vi "Motors Bk.vi"(2 "Motors Visa Ref":refnum<visa-resource-name>="COM7") -> ()   [LabVIEW 2010]
panel:
  in  "Cluster":T1
  in  "Y Speed (mm/s)":dbl=1.0 min=0.0
  in  "Delta Y (mm)":dbl=1.0
  in  "Theta Speed (deg/s)":dbl=1.0 min=0.0
  in  "Delta Theta (deg)":dbl=1.0
  in  "(mm/s)":dbl min=0.4
  in  "(mm/s) 3":dbl min=0.4
  in  "(mm/s) 2":dbl min=4.0
  in  "(degrees/s)":dbl min=8.0
  in  "X Set Slew Speed":bool
  in  "Y Set Slew Speed":bool
  in  "Z Set Slew Speed":bool
  in  "Theta Set Slew Speed":bool
  in  "Go To Saved Position":bool
  in  "Defined Positions":i32(listbox)
  in  "Steps to deactivate hard limit after finding datums":dbl=500.0
  out "Loop i":i32
types:
  T1 = cluster{"Stop X?":refnum<vi>, "Stop Y?":refnum<vi>, "Stop Z?":refnum<vi>, "Stop Theta?":refnum<vi>, "Backlash?":refnum<vi>, "Backlash X":refnum<vi>, "Backlash Y":refnum<vi>, "Backlash Z":refnum<vi>, "Backlash Theta":refnum<vi>, "Manual IO?":refnum<vi>, "Manual Communication is Active\n(Close Before Ending Program)":refnum<vi>, "Reset Motors?":refnum<vi>, "Set Jogger?":refnum<vi>, "Normal":refnum<vi>, "Fast":refnum<vi>, "Jogger Axis":refnum<vi>, "Redefine Origin as Current Location?":refnum<vi>, "Save Current Motor Parameters?":refnum<vi>, "Find Datums Nearest Hard Limits?":refnum<vi>, "Saved Limits":refnum<vi>, "Use Datums Nearest Hard Limits to Reset Origin?":refnum<vi>, "X Go?":refnum<vi>, "Y Go?":refnum<vi>, "Z Go?":refnum<vi>, "Theta Go?":refnum<vi>, "Jog-Mode":refnum<vi>, "x+?":refnum<vi>, "x-?":refnum<vi>, "y+?":refnum<vi>, "y-?":refnum<vi>, "z+?":refnum<vi>, "z-?":refnum<vi>, "theta+?":refnum<vi>, "theta-?":refnum<vi>, "X Set Slew Speed?":refnum<vi>, "(mm/s)":refnum<vi>, "Y Set Slew Speed?":refnum<vi>, "(mm/s)":refnum<vi>, "Z Set Slew Speed?":refnum<vi>, "(mm/s)":refnum<vi>, "Theta Set Slew Speed?":refnum<vi>, "(degrees/s)":refnum<vi>, "Go To Saved Position?":refnum<vi>, "Defined Positions":refnum<vi>, "Need to Update Motor Parameters":refnum<vi>, "X Jogger Normal Speed":refnum<vi>, "X Jogger Fast Speed":refnum<vi>, "Y Jogger Normal Speed":refnum<vi>, "Y Jogger Fast Speed":refnum<vi>, "Z Jogger Normal Speed":refnum<vi>, "Z Jogger Fast Speed":refnum<vi>, "Theta Jogger Normal Speed":refnum<vi>, "Theta Jogger Fast Speed":refnum<vi>, "X Moving":refnum<vi>, "Y Moving":refnum<vi>, "Z Moving":refnum<vi>, "Theta Moving":refnum<vi>, "X Slew Speed (mm or degree/s)":refnum<vi>, "Y Slew Speed (mm or degree/s)":refnum<vi>, "Z Slew Speed (mm or degree/s)":refnum<vi>, "Theta Slew Speed (mm or degree/s)":refnum<vi>, "X-Axis (mm)":refnum<vi>, "Y-Axis (mm)":refnum<vi>, "Z-Axis (mm)":refnum<vi>, "Theta (deg)":refnum<vi>, "X Multiplier":refnum<vi>, "Y Multiplier":refnum<vi>, "Z Multiplier":refnum<vi>, "Theta Multiplier":refnum<vi>, "Motors Online":refnum<vi>, "Motors Status":refnum<vi>, "Status X":refnum<vi>, "Status Y":refnum<vi>, "Status Z":refnum<vi>, "Status Theta":refnum<vi>, "Motors error":refnum<vi>, "QUIT":refnum<vi>, "EMERGENCY":refnum<vi>, "X Go To":refnum<vi>, "Y Go To":refnum<vi>, "Z Go To":refnum<vi>, "Theta Go To":refnum<vi>, "Delta X (mm)":refnum<vi>, "Delta Y (mm)":refnum<vi>, "Delta Z (mm)":refnum<vi>, "Delta Theta (deg)":refnum<vi>, "X Speed (mm/s)":refnum<vi>, "Y Speed (mm/s)":refnum<vi>, "Z Speed (mm/s)":refnum<vi>, "Theta Speed (deg/s)":refnum<vi>, "x+":refnum<vi>, "x-":refnum<vi>, "y+":refnum<vi>, "y-":refnum<vi>, "z+":refnum<vi>, "z-":refnum<vi>, "theta+":refnum<vi>, "theta-":refnum<vi>}
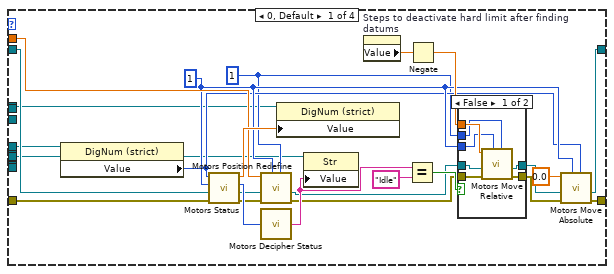
[diagram p4: hidden frame]
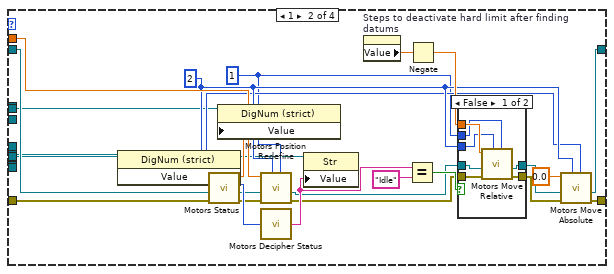
[diagram p6: hidden frame]
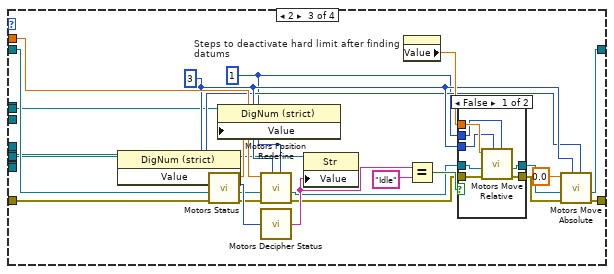
[diagram p8: hidden frame]
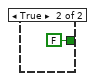
[diagram p12: hidden frame]
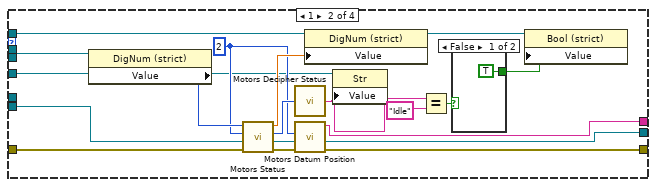
[diagram p13: hidden frame]
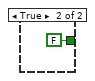
[diagram p14: hidden frame]
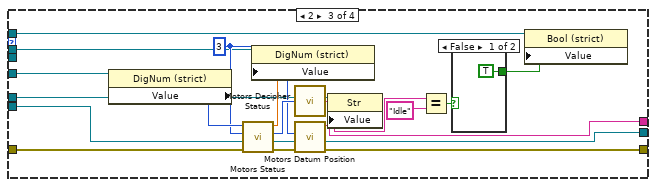
[diagram p15: hidden frame]
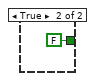
[diagram p16: hidden frame]
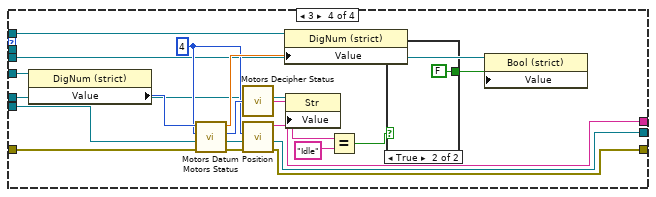
[diagram p17: hidden frame]
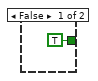
[diagram p18: hidden frame]
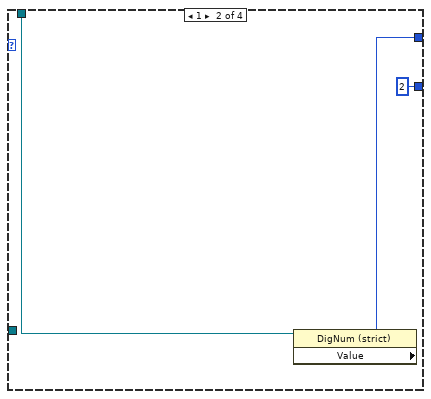
[diagram p19: hidden frame]
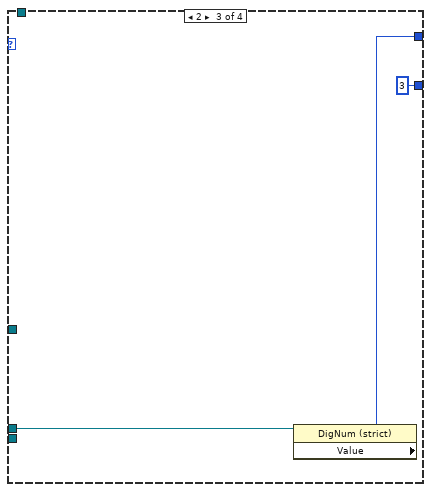
[diagram p20: hidden frame]
diagram:
  n1 = Unbundle("Cluster") -> ("Stop X?"=w69:refnum<vi>, "Stop Y?"=w68:refnum<vi>, "Stop Z?"=w67:refnum<vi>, "Stop Theta?"=w66:refnum<vi>, "Backlash?"=w65:refnum<vi>, "Backlash X"=w64:refnum<vi>, "Backlash Y"=w63:refnum<vi>, "Backlash Z"=w62:refnum<vi>, "Backlash Theta"=w61:refnum<vi>, "Manual IO?"=w60:refnum<vi>, "Manual Communication is Active\n(Close Before Ending Program)"=w53:refnum<vi>, "Reset Motors?"=w51:refnum<vi>, "Set Jogger?"=w50:refnum<vi>, "Normal"=w48:refnum<vi>, "Fast"=w47:refnum<vi>, "Jogger Axis"=w49:refnum<vi>, "Redefine Origin as Current Location?"=w46:refnum<vi>, "Save Current Motor Parameters?"=w45:refnum<vi>, "Find Datums Nearest Hard Limits?"=w44:refnum<vi>, "Saved Limits"=w43:refnum<vi>, "Use Datums Nearest Hard Limits to Reset Origin?"=w42:refnum<vi>, "X Go?"=w32:refnum<vi>, "Y Go?"=w29:refnum<vi>, "Z Go?"=w28:refnum<vi>, "Theta Go?"=w25:refnum<vi>, "Jog-Mode"=w22:refnum<vi>, "x+?"=w14:refnum<vi>, "x-?"=w15:refnum<vi>, "y+?"=w13:refnum<vi>, "y-?"=w12:refnum<vi>, "Need to Update Motor Parameters"=w34:refnum<vi>, "X Moving"=w21:refnum<vi>, "Y Moving"=w3:refnum<vi>, "Z Moving"=w41:refnum<vi>, "Theta Moving"=w40:refnum<vi>, "X-Axis (mm)"=w17:refnum<vi>, "Y-Axis (mm)"=w10:refnum<vi>, "Z-Axis (mm)"=w39:refnum<vi>, "Theta (deg)"=w37:refnum<vi>, "X Multiplier"=w19:refnum<vi>, "Y Multiplier"=w1:refnum<vi>, "Z Multiplier"=w27:refnum<vi>, "Theta Multiplier"=w24:refnum<vi>, "Motors Online"=w54:refnum<vi>, "Motors Status"=w56:refnum<vi>, "Status X"=w16:refnum<vi>, "Status Y"=w4:refnum<vi>, "Status Z"=w38:refnum<vi>, "Status Theta"=w36:refnum<vi>, "Motors error"=w59:refnum<vi>, "QUIT"=w58:refnum<vi>, "EMERGENCY"=w52:refnum<vi>, "X Go To"=w31:refnum<vi>, "Y Go To"=w30:refnum<vi>, "Z Go To"=w26:refnum<vi>, "Theta Go To"=w23:refnum<vi>, "Delta X (mm)"=w20:refnum<vi>, "Delta Y (mm)"=w2:refnum<vi>, "X Speed (mm/s)"=w18:refnum<vi>, "Y Speed (mm/s)"=w11:refnum<vi>, "x+"=w8:refnum<vi>, "x-"=w7:refnum<vi>, "y+"=w6:refnum<vi>, "y-"=w5:refnum<vi>)  [unwired: 34 out]
  n2 = property on="Property Node" class="Bool (strict)"(reference=w34, "Value"=TRUE) -> (reference out=w35:refnum<vi>)  [unwired: 1 in, 1 out]
  n3 = call "Motors Open.vi"("VISA in"="Motors Visa Ref") -> ("error out"=w73:errorcluster, "VISA out"=w70:refnum<visa-resource-name>)  [unwired: 1 in]
  n4 = call <vilib>:"Simple Error Handler.vi"("error in (no error)"=w73) -> ("error?"=w72:bool, "error out"=w74:errorcluster)  [unwired: 4 in, 3 out]
  n5 = property on="Property Node" class="Str"(reference=w56, "Value"="Opening Communications") -> (reference out=w57:refnum<vi>)  [unwired: 1 in, 1 out]
  n6 = property on="Property Node" class="Clust (strict)"(reference=w59, "Value"=w74) -> ()  [unwired: 1 in, 2 out]
  n7 = Not(x=w72) -> (.not. x?=w71:bool)
  n8 = case shown="True" w71 {
    tunnel: w57 -> [_ w164]
    tunnel: w70 -> [_ w163]
    tunnel: w59 -> [_ w162]
    tunnel: w58 -> [_ w161]
    tunnel: w69 -> [_ w160]
    tunnel: w68 -> [_ w159]
    tunnel: w67 -> [_ w158]
    tunnel: w66 -> [_ w157]
    tunnel: w65 -> [_ w156]
    tunnel: w64 -> [_ w155]
    tunnel: w63 -> [_ w154]
    tunnel: w62 -> [_ w153]
    tunnel: w61 -> [_ w152]
    tunnel: w60 -> [_ w151]
    tunnel: w53 -> [_ w150]
    tunnel: w52 -> [_ w149]
    tunnel: w51 -> [_ w148]
    tunnel: w50 -> [_ w147]
    tunnel: w49 -> [_ w146]
    tunnel: w19 -> [_ w145]
    tunnel: w1 -> [_ w144]
    tunnel: w27 -> [_ w143]
    tunnel: w24 -> [_ w142]
    tunnel: w35 -> [_ w141]
    tunnel: w48 -> [_ w140]
    tunnel: w47 -> [_ w139]
    tunnel: w46 -> [_ w138]
    tunnel: w45 -> [_ w137]
    tunnel: w44 -> [_ w136]
    tunnel: w19 -> [_ w134]
    tunnel: w17 -> [_ w133]
    tunnel: w16 -> [_ w132]
    tunnel: w21 -> [_ w131]
    tunnel: w43 -> [_ w130]
    tunnel: w42 -> [_ w129]
    tunnel: w3 -> [_ w128]
    tunnel: w41 -> [_ w127]
    tunnel: w40 -> [_ w126]
    tunnel: w19 -> [_ w125]
    tunnel: w1 -> [_ w124]
    tunnel: w27 -> [_ w123]
    tunnel: w24 -> [_ w122]
    tunnel: w17 -> [_ w121]
    tunnel: w10 -> [_ w120]
    tunnel: w39 -> [_ w119]
    tunnel: w16 -> [_ w118]
    tunnel: w4 -> [_ w117]
    tunnel: w38 -> [_ w116]
    tunnel: w37 -> [_ w115]
    tunnel: w36 -> [_ w114]
    tunnel: w32 -> [_ w113]
    tunnel: w19 -> [_ w112]
    tunnel: w31 -> [_ w111]
    tunnel: w1 -> [_ w110]
    tunnel: w30 -> [_ w109]
    tunnel: w29 -> [_ w108]
    tunnel: w28 -> [_ w107]
    tunnel: w27 -> [_ w106]
    tunnel: w26 -> [_ w105]
    tunnel: w25 -> [_ w104]
    tunnel: w24 -> [_ w103]
    tunnel: w23 -> [_ w102]
    tunnel: w15 -> [_ w101]
    tunnel: w22 -> [_ w100]
    tunnel: w21 -> [_ w99]
    tunnel: w20 -> [_ w98]
    tunnel: w19 -> [_ w97]
    tunnel: w18 -> [_ w96]
    tunnel: w17 -> [_ w95]
    tunnel: w14 -> [_ w94]
    tunnel: w15 -> [_ w93]
    tunnel: w16 -> [_ w92]
    tunnel: w15 -> [_ w91]
    tunnel: w14 -> [_ w90]
    tunnel: w14 -> [_ w89]
    tunnel: w13 -> [_ w88]
    tunnel: w12 -> [_ w87]
    tunnel: w1 -> [_ w86]
    tunnel: w11 -> [_ w85]
    tunnel: w10 -> [_ w84]
    tunnel: w8 -> [_ w83]
    tunnel: w7 -> [_ w82]
    tunnel: w6 -> [_ w81]
    tunnel: w5 -> [_ w80]
    tunnel: w4 -> [_ w79]
    tunnel: w3 -> [_ w78]
    tunnel: w2 -> [_ w77]
    tunnel: w1 -> [_ w76]
    frame False {
    }
    frame True {
      n9 = property on="Property Node" class="Str"(reference=w164, "Value"="Running") -> (reference out=w135:refnum<vi>)  [unwired: 1 in, 1 out]
      n10 = while {
        shift-right: _ -> [_]
        shift-left: w163 -> [w368]
        tunnel: w162 -> [w370]
        tunnel: w161 -> [w292]
        tunnel: w160 -> [w291]
        tunnel: w159 -> [w289]
        tunnel: w158 -> [w287]
        tunnel: w157 -> [w285]
        tunnel: w156 -> [w283]
        tunnel: w155 -> [w281]
        tunnel: w154 -> [w280]
        tunnel: w153 -> [w279]
        tunnel: w152 -> [w278]
        tunnel: w151 -> [w277]
        tunnel: w150 -> [w275]
        tunnel: w149 -> [w274]
        tunnel: w148 -> [w273]
        tunnel: w147 -> [w271]
        tunnel: w146 -> [w268]
        tunnel: w145 -> [w267]
        tunnel: w144 -> [w266]
        tunnel: w143 -> [w265]
        tunnel: w142 -> [w264]
        tunnel: w141 -> [w263]
        tunnel: w140 -> [w262]
        tunnel: w139 -> [w261]
        tunnel: w138 -> [w259]
        tunnel: w137 -> [w258]
        tunnel: w136 -> [w256]
        tunnel: w135 -> [w255]
        tunnel: w134 -> [w254]
        tunnel: w133 -> [w253]
        tunnel: w132 -> [w252]
        tunnel: w131 -> [w251]
        tunnel: w130 -> [w250]
        tunnel: w129 -> [w229]
        tunnel: w128 -> [w248]
        tunnel: w127 -> [w247]
        tunnel: w126 -> [w246]
        tunnel: w125 -> [w243]
        tunnel: w124 -> [w242]
        tunnel: w123 -> [w241]
        tunnel: w122 -> [w240]
        tunnel: w121 -> [w239]
        tunnel: w120 -> [w238]
        tunnel: w119 -> [w237]
        tunnel: w118 -> [w236]
        tunnel: w117 -> [w235]
        tunnel: w116 -> [w234]
        tunnel: w115 -> [w233]
        tunnel: w114 -> [w232]
        tunnel: w113 -> [w230]
        tunnel: w112 -> [w214]
        tunnel: w111 -> [w213]
        tunnel: w110 -> [w212]
        tunnel: w109 -> [w211]
        tunnel: w108 -> [w209]
        tunnel: w107 -> [w206]
        tunnel: w106 -> [w204]
        tunnel: w105 -> [w203]
        tunnel: w104 -> [w201]
        tunnel: w103 -> [w197]
        tunnel: w102 -> [w199]
        tunnel: w101 -> [w198]
        tunnel: w100 -> [w195]
        tunnel: w99 -> [w194]
        tunnel: w98 -> [w193]
        tunnel: w97 -> [w192]
        tunnel: w96 -> [w191]
        tunnel: w95 -> [w190]
        tunnel: w94 -> [w189]
        tunnel: w93 -> [w188]
        tunnel: w92 -> [w187]
        tunnel: w91 -> [w186]
        tunnel: w90 -> [w185]
        tunnel: w89 -> [w184]
        tunnel: w88 -> [w183]
        tunnel: w87 -> [w182]
        tunnel: w86 -> [w181]
        tunnel: w85 -> [w180]
        tunnel: w84 -> [w179]
        tunnel: w83 -> [w175]
        tunnel: w82 -> [w174]
        tunnel: w81 -> [w173]
        tunnel: w80 -> [w172]
        tunnel: w79 -> [w171]
        tunnel: w78 -> [w168]
        tunnel: w77 -> [w167]
        tunnel: w76 -> [w166]
        i -> [w293]
        stop <- w371 stop-if-true
        # "This loop contains all of the code that has to communicate directly with the manipulator motor controllers.  They are arranged linearly to ensure multiple serial I/O's are never attempted simultaneously.  Note that this loop executes very slowly (each serial I/O takes about 1/20 sec)."
        n11 = property on="Property Node" class="Bool (strict)"(reference=w183) -> (reference out=w169:refnum<vi>, "Value"=w307:bool)  [unwired: 1 in, 1 out]
        n12 = property on="Property Node" class="Bool (strict)"(reference=w182) -> (reference out=w170:refnum<vi>, "Value"=w308:bool)  [unwired: 1 in, 1 out]
        n13 = Or(x=w307, y=w308) -> (x .or. y?=w338:bool)
        n14 = property on="Property Node" class="Bool (strict)"(reference=w198) -> (reference out=w177:refnum<vi>, "Value"=w311:bool)  [unwired: 1 in, 1 out]
        n15 = property on="Property Node" class="Bool (strict)"(reference=w185) -> (reference out=w176:refnum<vi>, "Value"=w312:bool)  [unwired: 1 in, 1 out]
        n16 = property on="Property Node" class="Bool (strict)"(reference=w195) -> ("Value"=w196:bool)  [unwired: 1 in, 2 out]
        n17 = property on="Property Node" class="Bool (strict)"(reference=w230) -> (reference out=w178:refnum<vi>, "Value"=w231:bool)  [unwired: 1 in, 1 out]
        n18 = property on="Property Node" class="Bool (strict)"(reference=w292) -> ("Value"=w371:bool)  [unwired: 1 in, 2 out]
        n19 = Or(x=w312, y=w311) -> (x .or. y?=w344:bool)
        n20 = property on="Property Node" class="Bool (strict)"(reference=w291) -> (reference out=w215:refnum<vi>, "Value"=w290:bool)  [unwired: 1 in, 1 out]
        n21 = property on="Property Node" class="DigNum (strict)" props=["Value"]() -> ()  [unwired: 2 in, 3 out]
        n22 = property on="Property Node" class="Bool (strict)"(reference=w289) -> (reference out=w216:refnum<vi>, "Value"=w288:bool)  [unwired: 1 in, 1 out]
        n23 = property on="Property Node" class="Clust (strict)"(reference=w370) -> ("Value"=w369:errorcluster)  [unwired: 1 in, 2 out]
        n24 = property on="Property Node" class="Bool (strict)"(reference=w287) -> (reference out=w217:refnum<vi>, "Value"=w286:bool)  [unwired: 1 in, 1 out]
        n25 = property on="Property Node" class="Bool (strict)"(reference=w209) -> (reference out=w208:refnum<vi>, "Value"=w210:bool)  [unwired: 1 in, 1 out]
        n26 = case shown="True" w290 {
          tunnel: w369 -> [w1519 w1527]
          tunnel: w368 -> [w1520 w1526]
          tunnel: [w1520 w1524] -> w362
          tunnel: [w1519 w1523] -> w363
          tunnel: w215 -> [_ w1521]
          frame False {
          }
          frame True {
            n27 = call "Motors Stop.vi"("error in"=w1527, "Axis"=1, "VISA in"=w1526) -> ("error out"=w1523:errorcluster, "VISA out"=w1524:refnum<visa-resource-name>)
            n28 = property on="Property Node" class="Bool (strict)"(reference=w1521, "Value"=FALSE) -> ()  [unwired: 1 in, 2 out]
          }
        }
        n29 = property on="Property Node" class="Bool (strict)"(reference=w206) -> (reference out=w205:refnum<vi>, "Value"=w207:bool)  [unwired: 1 in, 1 out]
        n30 = case shown="True" w288 {
          tunnel: w363 -> [w1510 w1518]
          tunnel: w362 -> [w1511 w1517]
          tunnel: [w1511 w1515] -> w364
          tunnel: [w1510 w1514] -> w365
          tunnel: w216 -> [_ w1512]
          frame False {
          }
          frame True {
            n31 = call "Motors Stop.vi"("error in"=w1518, "Axis"=2, "VISA in"=w1517) -> ("error out"=w1514:errorcluster, "VISA out"=w1515:refnum<visa-resource-name>)
            n32 = property on="Property Node" class="Bool (strict)"(reference=w1512, "Value"=FALSE) -> ()  [unwired: 1 in, 2 out]
          }
        }
        n33 = property on="Property Node" class="Bool (strict)"(reference=w285) -> (reference out=w218:refnum<vi>, "Value"=w284:bool)  [unwired: 1 in, 1 out]
        n34 = case shown="True" w286 {
          tunnel: w365 -> [w1501 w1509]
          tunnel: w364 -> [w1502 w1508]
          tunnel: [w1502 w1506] -> w366
          tunnel: [w1501 w1505] -> w367
          tunnel: w217 -> [_ w1503]
          frame False {
          }
          frame True {
            n35 = call "Motors Stop.vi"("error in"=w1509, "Axis"=3, "VISA in"=w1508) -> ("error out"=w1505:errorcluster, "VISA out"=w1506:refnum<visa-resource-name>)
            n36 = property on="Property Node" class="Bool (strict)"(reference=w1503, "Value"=FALSE) -> ()  [unwired: 1 in, 2 out]
          }
        }
        n37 = property on="Property Node" class="Bool (strict)"(reference=w283) -> (reference out=w219:refnum<vi>, "Value"=w282:bool)  [unwired: 1 in, 1 out]
        n38 = property on="Property Node" class="Bool (strict)"(reference=w201) -> (reference out=w200:refnum<vi>, "Value"=w202:bool)  [unwired: 1 in, 1 out]
        n39 = case shown="True" w284 {
          tunnel: w367 -> [w1492 w1500]
          tunnel: w366 -> [w1493 w1499]
          tunnel: [w1493 w1497] -> w360
          tunnel: [w1492 w1496] -> w361
          tunnel: w218 -> [_ w1494]
          frame False {
          }
          frame True {
            n40 = property on="Property Node" class="Bool (strict)"(reference=w1494, "Value"=FALSE) -> ()  [unwired: 1 in, 2 out]
            n41 = call "Motors Stop.vi"("error in"=w1500, "Axis"=4, "VISA in"=w1499) -> ("error out"=w1496:errorcluster, "VISA out"=w1497:refnum<visa-resource-name>)
          }
        }
        n42 = case shown="True" w282 {
          tunnel: w360 -> [w1477 w1491]
          tunnel: [w1477 w1490] -> w359
          tunnel: [w1476 w1489] -> w358
          tunnel: w361 -> [w1476 w1488]
          tunnel: w281 -> [_ w1487]
          tunnel: w280 -> [_ w1485]
          tunnel: w279 -> [_ w1483]
          tunnel: w278 -> [_ w1481]
          tunnel: w219 -> [_ w1478]
          frame False {
          }
          frame True {
            n43 = property on="Property Node" class="DigNum (strict)"(reference=w1483) -> ("Value"=w1482:u32)  [unwired: 1 in, 2 out]
            n44 = property on="Property Node" class="DigNum (strict)"(reference=w1485) -> ("Value"=w1484:u32)  [unwired: 1 in, 2 out]
            n45 = property on="Property Node" class="DigNum (strict)"(reference=w1487) -> ("Value"=w1486:u32)  [unwired: 1 in, 2 out]
            n46 = property on="Property Node" class="Bool (strict)"(reference=w1478, "Value"=FALSE) -> ()  [unwired: 1 in, 2 out]
            n47 = property on="Property Node" class="DigNum (strict)"(reference=w1481) -> ("Value"=w1480:u32)  [unwired: 1 in, 2 out]
            n48 = call "Motors Backlash.vi"("X"=w1486, "Y"=w1484, "VISA in"=w1491, "error in"=w1488, "Z"=w1482, "Theta"=w1480) -> ("VISA out"=w1490:refnum<visa-resource-name>, "error out"=w1489:errorcluster)  [unwired: 2 in]
          }
        }
        n49 = property on="Property Node" class="Bool (strict)"(reference=w277) -> (reference out=w220:refnum<vi>, "Value"=w276:bool)  [unwired: 1 in, 1 out]
        n50 = case shown="True" w276 {
          tunnel: w359 -> [w1445 w1460]
          tunnel: w358 -> [w1446 w1459]
          tunnel: [w1446 w1458] -> w356
          tunnel: [w1445 w1457] -> w357
          tunnel: w274 -> [_ w1452]
          tunnel: w275 -> [_ w1451]
          tunnel: w220 -> [_ w1447]
          frame False {
          }
          frame True {
            n51 = flat-sequence {
              tunnel: w1459 -> [w1464]
              tunnel: w1460 -> [w1465]
              tunnel: [w1465] -> w1454
              tunnel: [w1464] -> w1453
              tunnel: w1451 -> [w1462]
              tunnel: [w1461] -> w1449
              tunnel: [w1469] -> w1456
              tunnel: [w1468] -> w1455
              tunnel: w1454 -> [w1471]
              tunnel: w1453 -> [w1470]
              tunnel: w1452 -> [w1467]
              tunnel: [w1466] -> w1450
              tunnel: w1449 -> [w1466]
              tunnel: [w1474] -> w1457
              tunnel: [w1475] -> w1458
              tunnel: w1456 -> [w1475]
              tunnel: w1455 -> [w1474]
              tunnel: w1450 -> [w1472]
              frame #0 {
                n52 = property on="Property Node" class="Bool (strict)"(reference=w1462, "Value"=TRUE ("Manual Communication is Active\n(Close Before Ending Program) 2")) -> (reference out=w1461:refnum<vi>)  [unwired: 1 in, 1 out]
              }
              frame #1 {
                n53 = call "Motors Manual IO.vi"("error in"=w1470, "Emergency Stop Reference"=w1467, "VISA in"=w1471) -> ("error out"=w1469:errorcluster, "VISA out"=w1468:refnum<visa-resource-name>)
              }
              frame #2 {
                n54 = property on="Property Node" class="Bool (strict)"(reference=w1472, "Value"=FALSE ("Manual Communication is Active\n(Close Before Ending Program)")) -> ()  [unwired: 1 in, 2 out]
              }
            }
            n55 = property on="Property Node" class="Bool (strict)"(reference=w1447, "Value"=FALSE) -> ()  [unwired: 1 in, 2 out]
          }
        }
        n56 = property on="Property Node" class="Ring (strict)"(reference=w268) -> ("Value"=w269:u16)  [unwired: 1 in, 2 out]
        n57 = property on="Property Node" class="Bool (strict)"(reference=w273) -> (reference out=w221:refnum<vi>, "Value"=w272:bool)  [unwired: 1 in, 1 out]
        n58 = case shown="True" w272 {
          tunnel: [w1437 w1444] -> w294
          tunnel: [w1438 w1443] -> w295
          tunnel: w357 -> [w1438 w1442]
          tunnel: w356 -> [w1437 w1441]
          tunnel: w221 -> [_ w1439]
          frame False {
          }
          frame True {
            n59 = call "Motors Reset.vi"("error in"=w1441, "VISA in"=w1442) -> ("error out"=w1444:errorcluster, "VISA out"=w1443:refnum<visa-resource-name>)
            n60 = property on="Property Node" class="Bool (strict)"(reference=w1439, "Value"=FALSE) -> ()  [unwired: 1 in, 2 out]
          }
        }
        n61 = property on="Property Node" class="Bool (strict)"() -> ("Value"=w309:bool)  [unwired: 2 in, 2 out]
        n62 = property on="Property Node" class="Bool (strict)"() -> ("Value"=w310:bool)  [unwired: 2 in, 2 out]
        n63 = case shown="0, Default" w269 {
          tunnel: [u32 1 u32 2 u32 3 u32 4] -> w304
          tunnel: [w776 w779 w782 w785] -> w303
          tunnel: w267 -> [w775 _ _ _]
          tunnel: w266 -> [_ w778 _ _]
          tunnel: w265 -> [_ _ w781 _]
          tunnel: w264 -> [_ _ _ w784]
          frame 0, Default {
            n64 = property on="Property Node" class="DigNum (strict)"(reference=w775) -> ("Value"=w776:u32)  [unwired: 1 in, 2 out]
          }
          frame 1 {
            n65 = property on="Property Node" class="DigNum (strict)"(reference=w778) -> ("Value"=w779:u32)  [unwired: 1 in, 2 out]
          }
          frame 2 {
            n66 = property on="Property Node" class="DigNum (strict)"(reference=w781) -> ("Value"=w782:u32)  [unwired: 1 in, 2 out]
          }
          frame 3 {
            n67 = property on="Property Node" class="DigNum (strict)"(reference=w784) -> ("Value"=w785:u32)  [unwired: 1 in, 2 out]
          }
        }
        n68 = Or(x=w310, y=w309) -> (x .or. y?=w341:bool)
        n69 = property on="Property Node" class="Bool (strict)"(reference=w271) -> (reference out=w222:refnum<vi>, "Value"=w270:bool)  [unwired: 1 in, 1 out]
        n70 = case shown="True" w270 {
          tunnel: w295 -> [w1421 w1432]
          tunnel: w294 -> [w1422 w1436]
          tunnel: [w1422 w1435] -> w354
          tunnel: [w1421 w1431] -> w355
          tunnel: w304 -> [_ w1434]
          tunnel: w303 -> [_ w1433]
          tunnel: w263 -> [_ w1429]
          tunnel: w262 -> [_ w1427]
          tunnel: w261 -> [_ w1425]
          tunnel: w222 -> [_ w1423]
          frame False {
          }
          frame True {
            n71 = property on="Property Node" class="DigNum (strict)"(reference=w1427) -> ("Value"=w1428:dbl)  [unwired: 1 in, 2 out]
            n72 = property on="Property Node" class="DigNum (strict)"(reference=w1425) -> ("Value"=w1426:dbl)  [unwired: 1 in, 2 out]
            n73 = property on="Property Node" class="Bool (strict)"(reference=w1429, "Value"=TRUE ("Need to Update Motor Parameters")) -> ()  [unwired: 1 in, 2 out]
            n74 = call "Motors Jogger Speed.vi"("Axis Multiplier"=w1433, "Axis"=w1434, "error in"=w1436, "VISA in"=w1432, "Fast Speed (mm or degree/sec)"=w1426, "Normal Speed (mm or degree/sec)"=w1428) -> ("error out"=w1435:errorcluster, "VISA out"=w1431:refnum<visa-resource-name>)  [unwired: 4 in]
            n75 = property on="Property Node" class="Bool (strict)"(reference=w1423, "Value"=FALSE) -> ()  [unwired: 1 in, 2 out]
          }
        }
        n76 = property on="Property Node" class="Bool (strict)"(reference=w259) -> (reference out=w223:refnum<vi>, "Value"=w260:bool)  [unwired: 1 in, 1 out]
        n77 = property on="Property Node" class="Bool (strict)"(reference=w258) -> (reference out=w225:refnum<vi>, "Value"=w224:bool)  [unwired: 1 in, 1 out]
        n78 = case shown="True" w260 {
          tunnel: w355 -> [w1413 w1420]
          tunnel: w354 -> [w1414 w1416]
          tunnel: [w1414 w1418] -> w226
          tunnel: [w1413 w1419] -> w353
          tunnel: w223 -> [_ w1415]
          frame False {
          }
          frame True {
            n79 = property on="Property Node" class="Bool (strict)"(reference=w1415, "Value"=FALSE) -> ()  [unwired: 1 in, 2 out]
            n80 = call "Motors Redefine Origin.vi"("error in"=w1416, "VISA in"=w1420) -> ("error out"=w1418:errorcluster, "VISA out"=w1419:refnum<visa-resource-name>)
          }
        }
        n81 = property on="Property Node" class="Bool (strict)"(reference=w256) -> (reference out=w228:refnum<vi>, "Value"=w257:bool)  [unwired: 1 in, 1 out]
        n82 = case shown="True" w224 {
          tunnel: w226 -> [w1406 w1412]
          tunnel: [w1406 w1411] -> w301
          tunnel: w353 -> [w1405 w1410]
          tunnel: [w1405 w1409] -> w300
          tunnel: w225 -> [_ w1408]
          frame False {
          }
          frame True {
            n83 = property on="Property Node" class="Bool (strict)"(reference=w1408, "Value"=FALSE) -> ()  [unwired: 1 in, 2 out]
            n84 = call "Motors Save.vi"("error in"=w1412, "VISA in"=w1410) -> ("error out"=w1411:errorcluster, "VISA out"=w1409:refnum<visa-resource-name>)
          }
        }
        n85 = case shown="True" w257 {
          tunnel: w301 -> [w589 w620]
          tunnel: [w589 w618] -> w298
          tunnel: [w588 w619] -> w296
          tunnel: w300 -> [w588 w621]
          tunnel: w255 -> [w586 w613]
          tunnel: w254 -> [_ w610]
          tunnel: w253 -> [_ w609]
          tunnel: w252 -> [_ w608]
          tunnel: w251 -> [_ w607]
          tunnel: w250 -> [w587 w606]
          tunnel: w242 -> [_ w605]
          tunnel: w238 -> [_ w604]
          tunnel: w235 -> [_ w603]
          tunnel: w248 -> [_ w602]
          tunnel: w241 -> [_ w601]
          tunnel: w237 -> [_ w600]
          tunnel: w234 -> [_ w599]
          tunnel: w247 -> [_ w598]
          tunnel: w240 -> [_ w597]
          tunnel: w233 -> [_ w596]
          tunnel: w232 -> [_ w595]
          tunnel: w246 -> [_ w594]
          tunnel: [w587 w593] -> w245
          tunnel: [w586 w592] -> w244
          tunnel: w228 -> [_ w591]
          frame False {
          }
          frame True {
            n86 = flat-sequence {
              tunnel: w620 -> [w626]
              tunnel: w621 -> [w627]
              tunnel: [w627] -> w617
              tunnel: [w626] -> w616
              tunnel: w613 -> [w623]
              tunnel: [w622] -> w611
              tunnel: w617 -> [w663]
              tunnel: w616 -> [w662]
              tunnel: [w658] -> w615
              tunnel: [w657] -> w614
              tunnel: [w647] -> w612
              tunnel: w611 -> [w647]
              tunnel: w610 -> [w646]
              tunnel: w609 -> [w645]
              tunnel: w608 -> [w644]
              tunnel: w607 -> [w643]
              tunnel: w606 -> [w641]
              tunnel: w605 -> [w640]
              tunnel: w604 -> [w639]
              tunnel: w603 -> [w638]
              tunnel: w602 -> [w637]
              tunnel: w601 -> [w636]
              tunnel: w600 -> [w635]
              tunnel: w599 -> [w634]
              tunnel: w598 -> [w633]
              tunnel: w597 -> [w632]
              tunnel: w596 -> [w631]
              tunnel: w595 -> [w630]
              tunnel: w594 -> [w629]
              tunnel: [w628] -> w593
              tunnel: [w773] -> w618
              tunnel: [w774] -> w619
              tunnel: w615 -> [w774]
              tunnel: w614 -> [w773]
              tunnel: w612 -> [w771]
              tunnel: [w770] -> w592
              frame #0 {
                n87 = call <vilib>:"Set Busy.vi"("disable click? (T)"=FALSE) -> ()  [unwired: 9 in, 2 out]
                n88 = property on="Property Node" class="Str"(reference=w623, "Value"="Finding Datums Nearest Hard Limits\nThis May Take a Few Minutes" ("Status")) -> (reference out=w622:refnum<vi>)  [unwired: 1 in, 1 out]
              }
              frame #1 {
                n89 = call "Motors Find Datums.vi"("error in"=w662, "VISA in"=w663) -> ("error out"=w659:errorcluster, "VISA out"=w660:refnum<visa-resource-name>)
                n90 = for {
                  N: 4 -> [_]
                  shift-right: [w683] -> w657
                  shift-left: w659 -> [w684]
                  shift-right: [w682] -> w658
                  shift-left: w660 -> [w685]
                  tunnel: [w681] -> w649 mode=indexing
                  tunnel: w646 -> [w679]
                  tunnel: w645 -> [w678]
                  tunnel: w644 -> [w677]
                  tunnel: w643 -> [w676]
                  tunnel: w640 -> [w675]
                  tunnel: w639 -> [w674]
                  tunnel: w638 -> [w673]
                  tunnel: w637 -> [w672]
                  tunnel: w636 -> [w671]
                  tunnel: w635 -> [w670]
                  tunnel: w634 -> [w669]
                  tunnel: w633 -> [w668]
                  tunnel: w632 -> [w667]
                  tunnel: w631 -> [w666]
                  tunnel: w630 -> [w665]
                  tunnel: w629 -> [w664]
                  i -> [w680]
                  n91 = case shown="0, Default" w680 {
                    tunnel: w684 -> [w698 w719 w740 w761]
                    tunnel: w685 -> [w699 w720 w741 w762]
                    tunnel: [w692 w713 w733 w754] -> w683
                    tunnel: [w693 w714 w734 w755] -> w682
                    tunnel: [w690 w711 w737 w758] -> w681
                    tunnel: w679 -> [w689 _ _ _]
                    tunnel: w678 -> [w688 _ _ _]
                    tunnel: w677 -> [w687 _ _ _]
                    tunnel: w676 -> [w686 _ _ _]
                    tunnel: w675 -> [_ w710 _ _]
                    tunnel: w674 -> [_ w709 _ _]
                    tunnel: w673 -> [_ w708 _ _]
                    tunnel: w672 -> [_ w707 _ _]
                    tunnel: w671 -> [_ _ w731 _]
                    tunnel: w670 -> [_ _ w730 _]
                    tunnel: w669 -> [_ _ w729 _]
                    tunnel: w668 -> [_ _ w728 _]
                    tunnel: w667 -> [_ _ _ w752]
                    tunnel: w666 -> [_ _ _ w751]
                    tunnel: w665 -> [_ _ _ w750]
                    tunnel: w664 -> [_ _ _ w749]
                    frame 0, Default {
                      w691 = 1 ("Axis")
                      n92 = property on="Property Node" class="DigNum (strict)"(reference=w689) -> ("Value"=w697:u32)  [unwired: 1 in, 2 out]
                      n93 = call "Motors Status.vi"("error in"=w698, "VISA in"=w699, "Axis"=w691, "Axis Multiplier"=w697) -> ("error out"=w694:errorcluster, "VISA out"=w695:refnum<visa-resource-name>, "OS"=w704:i32, "Actual Position (mm or deg)"=w696:dbl)  [unwired: 3 in]
                      n94 = property on="Property Node" class="DigNum (strict)"(reference=w688, "Value"=w696) -> ()  [unwired: 1 in, 2 out]
                      n95 = call "Motors Decipher Status.vi"("OS"=w704) -> ("Status"=w703:string)
                      n96 = call "Motors Datum Position.vi"("error in"=w694, "VISA in"=w695, "Axis"=w691) -> ("error out"=w692:errorcluster, "VISA out"=w693:refnum<visa-resource-name>, "Datum Position (steps)"=w690:string)  [unwired: 5 in]
                      n97 = property on="Property Node" class="Str"(reference=w687, "Value"=w703) -> ()  [unwired: 1 in, 2 out]
                      n98 = Equal?(x=w703, y="Idle") -> (x = y?=w701:bool)
                      n99 = case shown="False" w701 {
                        tunnel: [TRUE FALSE] -> w700
                        frame False {
                        }
                        frame True {
                        }
                      }
                      n100 = property on="Property Node" class="Bool (strict)"(reference=w686, "Value"=w700) -> ()  [unwired: 1 in, 2 out]
                    }
                    frame 1 {
                      w712 = 2 ("Axis")
                      n101 = property on="Property Node" class="DigNum (strict)"(reference=w710) -> ("Value"=w718:u32)  [unwired: 1 in, 2 out]
                      n102 = call "Motors Status.vi"("error in"=w719, "VISA in"=w720, "Axis"=w712, "Axis Multiplier"=w718) -> ("error out"=w715:errorcluster, "VISA out"=w716:refnum<visa-resource-name>, "OS"=w725:i32, "Actual Position (mm or deg)"=w717:dbl)  [unwired: 3 in]
                      n103 = call "Motors Decipher Status.vi"("OS"=w725) -> ("Status"=w723:string)
                      n104 = call "Motors Datum Position.vi"("error in"=w715, "VISA in"=w716, "Axis"=w712) -> ("error out"=w713:errorcluster, "VISA out"=w714:refnum<visa-resource-name>, "Datum Position (steps)"=w711:string)  [unwired: 5 in]
                      n105 = property on="Property Node" class="DigNum (strict)"(reference=w709, "Value"=w717) -> ()  [unwired: 1 in, 2 out]
                      n106 = property on="Property Node" class="Str"(reference=w708, "Value"=w723) -> ()  [unwired: 1 in, 2 out]
                      n107 = Equal?(x=w723, y="Idle") -> (x = y?=w722:bool)
                      n108 = case shown="False" w722 {
                        tunnel: [TRUE FALSE] -> w721
                        frame False {
                        }
                        frame True {
                        }
                      }
                      n109 = property on="Property Node" class="Bool (strict)"(reference=w707, "Value"=w721) -> ()  [unwired: 1 in, 2 out]
                    }
                    frame 2 {
                      w732 = 3 ("Axis")
                      n110 = property on="Property Node" class="DigNum (strict)"(reference=w731) -> ("Value"=w739:u32)  [unwired: 1 in, 2 out]
                      n111 = call "Motors Status.vi"("error in"=w740, "VISA in"=w741, "Axis"=w732, "Axis Multiplier"=w739) -> ("error out"=w735:errorcluster, "VISA out"=w736:refnum<visa-resource-name>, "OS"=w746:i32, "Actual Position (mm or deg)"=w738:dbl)  [unwired: 3 in]
                      n112 = property on="Property Node" class="DigNum (strict)"(reference=w730, "Value"=w738) -> ()  [unwired: 1 in, 2 out]
                      n113 = call "Motors Decipher Status.vi"("OS"=w746) -> ("Status"=w744:string)
                      n114 = call "Motors Datum Position.vi"("error in"=w735, "VISA in"=w736, "Axis"=w732) -> ("error out"=w733:errorcluster, "VISA out"=w734:refnum<visa-resource-name>, "Datum Position (steps)"=w737:string)  [unwired: 5 in]
                      n115 = property on="Property Node" class="Str"(reference=w729, "Value"=w744) -> ()  [unwired: 1 in, 2 out]
                      n116 = Equal?(x=w744, y="Idle") -> (x = y?=w743:bool)
                      n117 = case shown="False" w743 {
                        tunnel: [TRUE FALSE] -> w742
                        frame False {
                        }
                        frame True {
                        }
                      }
                      n118 = property on="Property Node" class="Bool (strict)"(reference=w728, "Value"=w742) -> ()  [unwired: 1 in, 2 out]
                    }
                    frame 3 {
                      w753 = 4 ("Axis")
                      n119 = property on="Property Node" class="DigNum (strict)"(reference=w752) -> ("Value"=w760:u32)  [unwired: 1 in, 2 out]
                      n120 = call "Motors Status.vi"("error in"=w761, "VISA in"=w762, "Axis"=w753, "Axis Multiplier"=w760) -> ("error out"=w756:errorcluster, "VISA out"=w757:refnum<visa-resource-name>, "OS"=w767:i32, "Actual Position (mm or deg)"=w759:dbl)  [unwired: 3 in]
                      n121 = call "Motors Decipher Status.vi"("OS"=w767) -> ("Status"=w765:string)
                      n122 = call "Motors Datum Position.vi"("error in"=w756, "VISA in"=w757, "Axis"=w753) -> ("error out"=w754:errorcluster, "VISA out"=w755:refnum<visa-resource-name>, "Datum Position (steps)"=w758:string)  [unwired: 5 in]
                      n123 = property on="Property Node" class="DigNum (strict)"(reference=w751, "Value"=w759) -> ()  [unwired: 1 in, 2 out]
                      n124 = property on="Property Node" class="Str"(reference=w750, "Value"=w765) -> ()  [unwired: 1 in, 2 out]
                      n125 = Equal?(x=w765, y="Idle") -> (x = y?=w764:bool)
                      n126 = case shown="True" w764 {
                        tunnel: [TRUE FALSE] -> w763
                        frame False {
                        }
                        frame True {
                        }
                      }
                      n127 = property on="Property Node" class="Bool (strict)"(reference=w749, "Value"=w763) -> ()  [unwired: 1 in, 2 out]
                    }
                  }
                }
                n128 = Build Array (concatenate)("Limits", w649) -> (w648:string[])
                n129 = Initialize Array("", 0 ("dimension size"), 0 ("dimension size")) -> (w655:string[][])
                n130 = Build Array (concatenate)(w648, w655) -> (w653:string[][])
                n131 = property on="Property Node" class="Path"(reference=w641) -> (reference out=w628:refnum<vi>, "Value"=w642:path)  [unwired: 1 in, 1 out]
                n132 = Transpose 2D Array(2D array=w653) -> (transposed array=w652:string[][])
                n133 = call "Motors Position Rewrite.vi"("file path"=w642, "Array of Positions"=w652) -> ()  [unwired: 9 in]
              }
              frame #2 {
                n134 = call <vilib>:"Unset Busy.vi"() -> ()  [unwired: 11 in, 1 out]
                n135 = property on="Property Node" class="Str"(reference=w771, "Value"="Running" ("Status")) -> (reference out=w770:refnum<vi>)  [unwired: 1 in, 1 out]
              }
            }
            n136 = property on="Property Node" class="Bool (strict)"(reference=w591, "Value"=FALSE) -> ()  [unwired: 1 in, 2 out]
          }
        }
        n137 = property on="Property Node" class="Bool (strict)"(reference=w229) -> (reference out=w227:refnum<vi>, "Value"=w249:bool)  [unwired: 1 in, 1 out]
        n138 = case shown="True" w249 {
          tunnel: [w374 w395] -> w299
          tunnel: w298 -> [w374 w397]
          tunnel: [w373 w394] -> w297
          tunnel: w296 -> [w373 w398]
          tunnel: w245 -> [_ w393]
          tunnel: w244 -> [w372 w377]
          tunnel: w243 -> [_ w392]
          tunnel: w242 -> [_ w391]
          tunnel: w241 -> [_ w390]
          tunnel: w240 -> [_ w389]
          tunnel: w239 -> [_ w388]
          tunnel: w238 -> [_ w387]
          tunnel: w237 -> [_ w386]
          tunnel: w236 -> [_ w385]
          tunnel: w235 -> [_ w384]
          tunnel: w234 -> [_ w383]
          tunnel: w233 -> [_ w382]
          tunnel: w232 -> [_ w381]
          tunnel: [w372 w378] -> _
          tunnel: w227 -> [_ w376]
          frame False {
          }
          frame True {
            n139 = property on="Property Node" class="Bool (strict)"(reference=w376, "Value"=FALSE) -> ()  [unwired: 1 in, 2 out]
            n140 = flat-sequence {
              tunnel: w397 -> [w402]
              tunnel: [w402] -> w396
              tunnel: w377 -> [w400]
              tunnel: [w399] -> w379
              tunnel: w398 -> [w426]
              tunnel: w396 -> [w427]
              tunnel: [w422] -> w395
              tunnel: [w421] -> w394
              tunnel: w393 -> [w417]
              tunnel: w392 -> [w415]
              tunnel: w391 -> [w414]
              tunnel: w390 -> [w413]
              tunnel: w389 -> [w412]
              tunnel: w388 -> [w411]
              tunnel: w387 -> [w410]
              tunnel: w386 -> [w409]
              tunnel: w385 -> [w408]
              tunnel: w384 -> [w407]
              tunnel: w383 -> [w406]
              tunnel: w382 -> [w405]
              tunnel: w381 -> [w404]
              tunnel: [w403] -> w380
              tunnel: w379 -> [w403]
              tunnel: w380 -> [w584]
              tunnel: [w583] -> w378
              frame #0 {
                n141 = call <vilib>:"Set Busy.vi"() -> ()  [unwired: 10 in, 2 out]
                n142 = property on="Property Node" class="Str"(reference=w400, "Value"="Finding Datums Nearest Hard Limits\nThis May Take a Few Minutes" ("Status")) -> (reference out=w399:refnum<vi>)  [unwired: 1 in, 1 out]
              }
              frame #1 {
                n143 = property on="Property Node" class="Path"(reference=w417) -> ("Value"=w416:path)  [unwired: 1 in, 2 out]
                n144 = call "Motors Find Datums.vi"("error in"=w427, "VISA in"=w426) -> ("error out"=w424:errorcluster, "VISA out"=w425:refnum<visa-resource-name>)
                n145 = call "Motors Position Load.vi"("error in"=w424, "file path"=w416) -> ("error out"=w423:errorcluster, "Positions"=w420:string[][])
                n146 = Delete From Array(array=w420, index (row)=0) -> (array with subset deleted=w418:string[][])  [unwired: 2 in, 1 out]
                n147 = for {
                  shift-right: [w446] -> w422
                  shift-left: w423 -> [w447]
                  shift-right: [w445] -> w421
                  shift-left: w425 -> [w448]
                  tunnel: w418 -> [w444] mode=indexing
                  tunnel: w415 -> [w439]
                  tunnel: w414 -> [w438]
                  tunnel: w413 -> [w437]
                  tunnel: w412 -> [w436]
                  tunnel: w411 -> [w435]
                  tunnel: w410 -> [w434]
                  tunnel: w409 -> [w433]
                  tunnel: w408 -> [w432]
                  tunnel: w407 -> [w431]
                  tunnel: w406 -> [w430]
                  tunnel: w405 -> [w429]
                  tunnel: w404 -> [w428]
                  i -> [w441]
                  n148 = Index Array(array=w444, index=0) -> (element=w443:string)
                  n149 = Fract/Exp String To Number(string=w443) -> (number=w442:dbl)  [unwired: 3 in, 1 out]
                  n150 = case shown="3" w441 {
                    tunnel: w447 -> [w468 w502 w532 w568]
                    tunnel: w448 -> [w469 w503 w533 w569]
                    tunnel: [w462 w495 w524 w561] -> w446
                    tunnel: [w463 w496 w525 w562] -> w445
                    tunnel: w442 -> [w464 w498 w535 w564]
                    tunnel: w439 -> [w451 _ _ _]
                    tunnel: w438 -> [_ w485 _ _]
                    tunnel: w437 -> [_ _ w519 _]
                    tunnel: w436 -> [_ _ _ w552]
                    tunnel: w435 -> [w450 _ _ _]
                    tunnel: w434 -> [_ w484 _ _]
                    tunnel: w433 -> [_ _ w518 _]
                    tunnel: w432 -> [w449 _ _ _]
                    tunnel: w431 -> [_ w483 _ _]
                    tunnel: w430 -> [_ _ w517 _]
                    tunnel: w429 -> [_ _ _ w551]
                    tunnel: w428 -> [_ _ _ w550]
                    frame 0, Default {
                      w452 = u32 1 ("Axis Multiplier")
                      w454 = 1 ("Axis")
                      n151 = property on="Property Node" class="DigNum (strict)"(reference=w451) -> ("Value"=w453:u32)  [unwired: 1 in, 2 out]
                      n152 = call "Motors Status.vi"("error in"=w468, "VISA in"=w469, "Axis"=w454, "Axis Multiplier"=w453) -> ("error out"=w465:errorcluster, "VISA out"=w466:refnum<visa-resource-name>, "OS"=w473:i32, "Actual Position (mm or deg)"=w467:dbl)  [unwired: 3 in]
                      n153 = call "Motors Position Redefine.vi"("Axis Multiplier"=w452, "Axis"=w454, "error in"=w465, "VISA in"=w466, "Position (mm or deg)"=w464) -> ("error out"=w459:errorcluster, "VISA out"=w456:refnum<visa-resource-name>)  [unwired: 5 in]
                      n154 = call "Motors Decipher Status.vi"("OS"=w473) -> ("Status"=w472:string)
                      n155 = property on="Property Node" class="DigNum (strict)"(reference=w450, "Value"=w467) -> ()  [unwired: 1 in, 2 out]
                      n156 = property on="Property Node" class="Str"(reference=w449, "Value"=w472) -> ()  [unwired: 1 in, 2 out]
                      n157 = property on="Steps to deactivate hard limit after finding datums" class="DigNum (strict)"() -> ("Value"=w460:dbl)  [unwired: 2 in, 2 out]
                      n158 = Equal?(x=w472, y="Idle") -> (x = y?=w470:bool)
                      n159 = Negate(x=w460) -> (-x=w455:dbl)
                      n160 = case shown="False" w470 {
                        tunnel: w459 -> [w480 w482]
                        tunnel: [w479 w482] -> w458
                        tunnel: w456 -> [w478 w481]
                        tunnel: [w477 w481] -> w457
                        tunnel: w455 -> [w476 _]
                        tunnel: w454 -> [w475 _]
                        tunnel: w452 -> [w474 _]
                        frame False {
                          n161 = call "Motors Move Relative.vi"("Axis Multiplier"=w474, "Axis"=w475, "error in"=w480, "VISA in"=w478, "Distance (mm)"=w476) -> ("error out"=w479:errorcluster, "VISA out"=w477:refnum<visa-resource-name>)  [unwired: 5 in]
                        }
                        frame True {
                        }
                      }
                      n162 = call "Motors Move Absolute.vi"("Axis Multiplier"=w453, "Axis"=w454, "error in"=w458, "VISA in"=w457, "Position (mm or degree)"=0.0) -> ("error out"=w462:errorcluster, "VISA out"=w463:refnum<visa-resource-name>)  [unwired: 5 in]
                    }
                    frame 1 {
                      w486 = u32 1 ("Axis Multiplier")
                      w488 = 2 ("Axis")
                      n163 = property on="Property Node" class="DigNum (strict)"(reference=w485) -> ("Value"=w487:u32)  [unwired: 1 in, 2 out]
                      n164 = call "Motors Status.vi"("error in"=w502, "VISA in"=w503, "Axis"=w488, "Axis Multiplier"=w487) -> ("error out"=w499:errorcluster, "VISA out"=w500:refnum<visa-resource-name>, "OS"=w507:i32, "Actual Position (mm or deg)"=w501:dbl)  [unwired: 3 in]
                      n165 = property on="Property Node" class="DigNum (strict)"(reference=w484, "Value"=w501) -> ()  [unwired: 1 in, 2 out]
                      n166 = call "Motors Position Redefine.vi"("Axis Multiplier"=w486, "Axis"=w488, "error in"=w499, "VISA in"=w500, "Position (mm or deg)"=w498) -> ("error out"=w492:errorcluster, "VISA out"=w493:refnum<visa-resource-name>)  [unwired: 5 in]
                      n167 = call "Motors Decipher Status.vi"("OS"=w507) -> ("Status"=w505:string)
                      n168 = property on="Property Node" class="Str"(reference=w483, "Value"=w505) -> ()  [unwired: 1 in, 2 out]
                      n169 = property on="Steps to deactivate hard limit after finding datums" class="DigNum (strict)"() -> ("Value"=w494:dbl)  [unwired: 2 in, 2 out]
                      n170 = Equal?(x=w505, y="Idle") -> (x = y?=w504:bool)
                      n171 = Negate(x=w494) -> (-x=w489:dbl)
                      n172 = case shown="False" w504 {
                        tunnel: w493 -> [w514 w515]
                        tunnel: w492 -> [w513 w516]
                        tunnel: [w512 w515] -> w491
                        tunnel: [w511 w516] -> w490
                        tunnel: w489 -> [w510 _]
                        tunnel: w488 -> [w509 _]
                        tunnel: w486 -> [w508 _]
                        frame False {
                          n173 = call "Motors Move Relative.vi"("Axis Multiplier"=w508, "Axis"=w509, "error in"=w513, "VISA in"=w514, "Distance (mm)"=w510) -> ("error out"=w511:errorcluster, "VISA out"=w512:refnum<visa-resource-name>)  [unwired: 5 in]
                        }
                        frame True {
                        }
                      }
                      n174 = call "Motors Move Absolute.vi"("Axis Multiplier"=w487, "Axis"=w488, "error in"=w490, "VISA in"=w491, "Position (mm or degree)"=0.0) -> ("error out"=w495:errorcluster, "VISA out"=w496:refnum<visa-resource-name>)  [unwired: 5 in]
                    }
                    frame 2 {
                      w520 = u32 1 ("Axis Multiplier")
                      w522 = 3 ("Axis")
                      n175 = property on="Property Node" class="DigNum (strict)"(reference=w519) -> ("Value"=w521:u32)  [unwired: 1 in, 2 out]
                      n176 = call "Motors Status.vi"("error in"=w532, "VISA in"=w533, "Axis"=w522, "Axis Multiplier"=w521) -> ("error out"=w530:errorcluster, "VISA out"=w531:refnum<visa-resource-name>, "OS"=w540:i32, "Actual Position (mm or deg)"=w536:dbl)  [unwired: 3 in]
                      n177 = property on="Property Node" class="DigNum (strict)"(reference=w518, "Value"=w536) -> ()  [unwired: 1 in, 2 out]
                      n178 = call "Motors Position Redefine.vi"("Axis Multiplier"=w520, "Axis"=w522, "error in"=w530, "VISA in"=w531, "Position (mm or deg)"=w535) -> ("error out"=w528:errorcluster, "VISA out"=w529:refnum<visa-resource-name>)  [unwired: 5 in]
                      n179 = call "Motors Decipher Status.vi"("OS"=w540) -> ("Status"=w538:string)
                      n180 = property on="Property Node" class="Str"(reference=w517, "Value"=w538) -> ()  [unwired: 1 in, 2 out]
                      n181 = property on="Steps to deactivate hard limit after finding datums" class="DigNum (strict)"() -> ("Value"=w523:dbl)  [unwired: 2 in, 2 out]
                      n182 = Equal?(x=w538, y="Idle") -> (x = y?=w537:bool)
                      n183 = case shown="False" w537 {
                        tunnel: w529 -> [w547 w548]
                        tunnel: w528 -> [w546 w549]
                        tunnel: [w545 w548] -> w527
                        tunnel: [w544 w549] -> w526
                        tunnel: w523 -> [w543 _]
                        tunnel: w522 -> [w542 _]
                        tunnel: w520 -> [w541 _]
                        frame False {
                          n184 = call "Motors Move Relative.vi"("Axis Multiplier"=w541, "Axis"=w542, "error in"=w546, "VISA in"=w547, "Distance (mm)"=w543) -> ("error out"=w544:errorcluster, "VISA out"=w545:refnum<visa-resource-name>)  [unwired: 5 in]
                        }
                        frame True {
                        }
                      }
                      n185 = call "Motors Move Absolute.vi"("Axis Multiplier"=w521, "Axis"=w522, "error in"=w526, "VISA in"=w527, "Position (mm or degree)"=0.0) -> ("error out"=w524:errorcluster, "VISA out"=w525:refnum<visa-resource-name>)  [unwired: 5 in]
                    }
                    frame 3 {
                      w553 = u32 1 ("Axis Multiplier")
                      w555 = 4 ("Axis")
                      n186 = property on="Property Node" class="DigNum (strict)"(reference=w552) -> ("Value"=w554:u32)  [unwired: 1 in, 2 out]
                      n187 = call "Motors Status.vi"("error in"=w568, "VISA in"=w569, "Axis"=w555, "Axis Multiplier"=w554) -> ("error out"=w565:errorcluster, "VISA out"=w566:refnum<visa-resource-name>, "OS"=w573:i32, "Actual Position (mm or deg)"=w567:dbl)  [unwired: 3 in]
                      n188 = property on="Property Node" class="DigNum (strict)"(reference=w551, "Value"=w567) -> ()  [unwired: 1 in, 2 out]
                      n189 = call "Motors Position Redefine.vi"("Axis Multiplier"=w553, "Axis"=w555, "error in"=w565, "VISA in"=w566, "Position (mm or deg)"=w564) -> ("error out"=w559:errorcluster, "VISA out"=w560:refnum<visa-resource-name>)  [unwired: 5 in]
                      n190 = call "Motors Decipher Status.vi"("OS"=w573) -> ("Status"=w571:string)
                      n191 = property on="Property Node" class="Str"(reference=w550, "Value"=w571) -> ()  [unwired: 1 in, 2 out]
                      n192 = Equal?(x=w571, y="Idle") -> (x = y?=w570:bool)
                      n193 = case shown="False" w570 {
                        tunnel: w560 -> [w580 w582]
                        tunnel: w559 -> [w579 w581]
                        tunnel: [w578 w582] -> w558
                        tunnel: [w577 w581] -> w557
                        tunnel: "Steps to deactivate hard limit after finding datums" -> [w576 _]
                        tunnel: w555 -> [w575 _]
                        tunnel: w553 -> [w574 _]
                        frame False {
                          n194 = call "Motors Move Relative.vi"("Axis Multiplier"=w574, "Axis"=w575, "error in"=w579, "VISA in"=w580, "Distance (mm)"=w576) -> ("error out"=w577:errorcluster, "VISA out"=w578:refnum<visa-resource-name>)  [unwired: 5 in]
                        }
                        frame True {
                        }
                      }
                      n195 = call "Motors Move Absolute.vi"("Axis Multiplier"=w554, "Axis"=w555, "error in"=w557, "VISA in"=w558, "Position (mm or degree)"=0.0) -> ("error out"=w561:errorcluster, "VISA out"=w562:refnum<visa-resource-name>)  [unwired: 5 in]
                    }
                  }
                }
              }
              frame #2 {
                n196 = call <vilib>:"Unset Busy.vi"() -> ()  [unwired: 11 in, 1 out]
                n197 = property on="Property Node" class="Str"(reference=w584, "Value"="Running" ("Status")) -> (reference out=w583:refnum<vi>)  [unwired: 1 in, 1 out]
              }
            }
          }
        }
        n198 = case shown="True" w231 {
          tunnel: w297 -> [w1393 w1401]
          tunnel: w299 -> [w1392 w1404]
          tunnel: [w1393 w1402] -> w352
          tunnel: [w1392 w1403] -> w351
          tunnel: w178 -> [_ w1399]
          tunnel: w214 -> [_ w1396]
          tunnel: w213 -> [_ w1394]
          frame False {
          }
          frame True {
            n199 = property on="Property Node" class="DigNum (strict)"(reference=w1396) -> ("Value"=w1397:u32)  [unwired: 1 in, 2 out]
            n200 = property on="Property Node" class="DigNum (strict)"(reference=w1394) -> ("Value"=w1395:dbl)  [unwired: 1 in, 2 out]
            n201 = property on="Property Node" class="Bool (strict)"(reference=w1399, "Value"=FALSE) -> ()  [unwired: 1 in, 2 out]
            n202 = call "Motors Move Absolute.vi"("Axis Multiplier"=w1397, "Axis"=u32 1, "error in"=w1404, "VISA in"=w1401, "Position (mm or degree)"=w1395) -> ("error out"=w1403:errorcluster, "VISA out"=w1402:refnum<visa-resource-name>)  [unwired: 5 in]
          }
        }
        n203 = case shown="True" w210 {
          tunnel: w352 -> [w1380 w1388]
          tunnel: w351 -> [w1379 w1391]
          tunnel: [w1380 w1389] -> w350
          tunnel: [w1379 w1390] -> w349
          tunnel: w212 -> [_ w1384]
          tunnel: w211 -> [_ w1383]
          tunnel: w208 -> [_ w1381]
          frame False {
          }
          frame True {
            n204 = property on="Property Node" class="DigNum (strict)"(reference=w1384) -> ("Value"=w1386:u32)  [unwired: 1 in, 2 out]
            n205 = property on="Property Node" class="DigNum (strict)"(reference=w1383) -> ("Value"=w1385:dbl)  [unwired: 1 in, 2 out]
            n206 = property on="Property Node" class="Bool (strict)"(reference=w1381, "Value"=FALSE) -> ()  [unwired: 1 in, 2 out]
            n207 = call "Motors Move Absolute.vi"("Axis Multiplier"=w1386, "Axis"=u32 2, "error in"=w1391, "VISA in"=w1388, "Position (mm or degree)"=w1385) -> ("error out"=w1390:errorcluster, "VISA out"=w1389:refnum<visa-resource-name>)  [unwired: 5 in]
          }
        }
        n208 = case shown="True" w207 {
          tunnel: w350 -> [w1367 w1373]
          tunnel: w349 -> [w1366 w1378]
          tunnel: [w1367 w1376] -> w348
          tunnel: [w1366 w1377] -> w347
          tunnel: w205 -> [_ w1370]
          tunnel: w204 -> [_ w1369]
          tunnel: w203 -> [_ w1368]
          frame False {
          }
          frame True {
            n209 = property on="Property Node" class="DigNum (strict)"(reference=w1369) -> ("Value"=w1374:u32)  [unwired: 1 in, 2 out]
            n210 = property on="Property Node" class="DigNum (strict)"(reference=w1368) -> ("Value"=w1372:dbl)  [unwired: 1 in, 2 out]
            n211 = property on="Property Node" class="Bool (strict)"(reference=w1370, "Value"=FALSE) -> ()  [unwired: 1 in, 2 out]
            n212 = call "Motors Move Absolute.vi"("Axis Multiplier"=w1374, "Axis"=u32 3, "error in"=w1378, "VISA in"=w1373, "Position (mm or degree)"=w1372) -> ("error out"=w1377:errorcluster, "VISA out"=w1376:refnum<visa-resource-name>)  [unwired: 5 in]
          }
        }
        n213 = case shown="True" w202 {
          tunnel: w348 -> [w1353 w1362]
          tunnel: w347 -> [w1354 w1365]
          tunnel: [w1354 w1364] -> w345
          tunnel: [w1353 w1363] -> w346
          tunnel: w200 -> [_ w1357]
          tunnel: w197 -> [_ w1356]
          tunnel: w199 -> [_ w1355]
          frame False {
          }
          frame True {
            n214 = property on="Property Node" class="DigNum (strict)"(reference=w1355) -> ("Value"=w1359:dbl)  [unwired: 1 in, 2 out]
            n215 = property on="Property Node" class="DigNum (strict)"(reference=w1356) -> ("Value"=w1360:u32)  [unwired: 1 in, 2 out]
            n216 = property on="Property Node" class="Bool (strict)"(reference=w1357, "Value"=FALSE) -> ()  [unwired: 1 in, 2 out]
            n217 = call "Motors Move Absolute.vi"("Axis Multiplier"=w1360, "Axis"=u32 4, "error in"=w1365, "VISA in"=w1362, "Position (mm or degree)"=w1359) -> ("error out"=w1364:errorcluster, "VISA out"=w1363:refnum<visa-resource-name>)  [unwired: 5 in]
          }
        }
        n218 = case shown="True" w344 {
          tunnel: w346 -> [w1235 w1258]
          tunnel: w345 -> [w1234 w1257]
          tunnel: w196 -> [_ w1259]
          tunnel: [w1235 w1255] -> w343
          tunnel: [w1234 w1254] -> w342
          tunnel: w311 -> [_ w1256]
          tunnel: w194 -> [_ w1251]
          tunnel: w193 -> [_ w1250]
          tunnel: w192 -> [_ w1249]
          tunnel: w192 -> [_ w1248]
          tunnel: w191 -> [_ w1247]
          tunnel: w190 -> [_ w1246]
          tunnel: w189 -> [_ w1245]
          tunnel: w188 -> [_ w1244]
          tunnel: w187 -> [_ w1243]
          tunnel: w186 -> [_ w1242]
          tunnel: w185 -> [_ w1241]
          tunnel: w184 -> [_ w1240]
          tunnel: w177 -> [_ w1239]
          tunnel: w176 -> [_ w1238]
          tunnel: w175 -> [_ w1237]
          tunnel: w174 -> [_ w1236]
          frame False {
          }
          frame True {
            n219 = flat-sequence {
              tunnel: w1259 -> [w1276]
              tunnel: w1258 -> [w1275]
              tunnel: w1257 -> [w1274]
              tunnel: w1256 -> [w1273]
              tunnel: [w1272] -> w1253
              tunnel: [w1271] -> w1252
              tunnel: w1251 -> [w1270]
              tunnel: w1250 -> [w1269]
              tunnel: w1249 -> [w1268]
              tunnel: w1248 -> [w1267]
              tunnel: w1247 -> [w1266]
              tunnel: w1246 -> [w1265]
              tunnel: w1245 -> [w1264]
              tunnel: w1244 -> [w1263]
              tunnel: w1243 -> [w1262]
              tunnel: w1237 -> [w1261]
              tunnel: w1236 -> [w1260]
              tunnel: [w1351] -> w1254
              tunnel: [w1352] -> w1255
              tunnel: w1253 -> [w1352]
              tunnel: w1252 -> [w1351]
              tunnel: w1242 -> [_]
              tunnel: w1241 -> [_]
              tunnel: w1240 -> [_]
              tunnel: w1239 -> [w1348]
              tunnel: w1238 -> [w1347]
              frame #0 {
                n220 = case shown="True" w1276 {
                  tunnel: w1275 -> [w1286 w1318]
                  tunnel: w1274 -> [w1282 w1321]
                  tunnel: w1273 -> [w1285 w1326]
                  tunnel: [w1284 w1323] -> w1272
                  tunnel: [w1283 w1322] -> w1271
                  tunnel: w1270 -> [w1280 _]
                  tunnel: w1269 -> [w1278 _]
                  tunnel: w1268 -> [w1277 _]
                  tunnel: w1267 -> [_ w1314]
                  tunnel: w1266 -> [_ w1312]
                  tunnel: w1265 -> [_ w1311]
                  tunnel: w1264 -> [_ w1310]
                  tunnel: w1263 -> [_ w1309]
                  tunnel: w1262 -> [_ w1308]
                  tunnel: w1261 -> [_ w1307]
                  tunnel: w1260 -> [_ w1306]
                  frame False {
                    n221 = property on="Property Node" class="Bool (strict)"(reference=w1280) -> (reference out=w1279:refnum<vi>, "Value"=w1281:bool)  [unwired: 1 in, 1 out]
                    n222 = case shown="False" w1281 {
                      tunnel: w1286 -> [w1294 w1305]
                      tunnel: w1282 -> [w1299 w1304]
                      tunnel: w1285 -> [w1298 _]
                      tunnel: [w1296 w1305] -> w1284
                      tunnel: [w1297 w1304] -> w1283
                      tunnel: w1279 -> [w1290 _]
                      tunnel: w1278 -> [w1288 _]
                      tunnel: w1277 -> [w1287 _]
                      frame False {
                        n223 = property on="Property Node" class="DigNum (strict)"(reference=w1288) -> ("Value"=w1289:dbl)  [unwired: 1 in, 2 out]
                        n224 = property on="Property Node" class="Bool (strict)"(reference=w1290, "Value"=TRUE ("X Moving")) -> ()  [unwired: 1 in, 2 out]
                        n225 = case shown="True" w1298 {
                          tunnel: w1289 -> [w1300 w1302]
                          tunnel: [w1300 w1301] -> w1295
                          frame False {
                          }
                          frame True {
                            n226 = Multiply(x=w1302, y=-1.0) -> (x*y=w1301:dbl)
                          }
                        }
                        n227 = property on="Property Node" class="DigNum (strict)"(reference=w1287) -> ("Value"=w1292:u32)  [unwired: 1 in, 2 out]
                        n228 = call "Motors Move Relative.vi"("Axis Multiplier"=w1292, "Axis"=1, "error in"=w1299, "VISA in"=w1294, "Distance (mm)"=w1295) -> ("error out"=w1297:errorcluster, "VISA out"=w1296:refnum<visa-resource-name>)  [unwired: 5 in]
                      }
                      frame True {
                      }
                    }
                  }
                  frame True {
                    w1315 = 1 ("Axis")
                    n229 = property on="Property Node" class="DigNum (strict)"(reference=w1312) -> ("Value"=w1313:dbl)  [unwired: 1 in, 2 out]
                    n230 = property on="Property Node" class="DigNum (strict)"(reference=w1314) -> ("Value"=w1316:u32)  [unwired: 1 in, 2 out]
                    n231 = case shown="True" w1326 {
                      tunnel: w1313 -> [w1343 w1345]
                      tunnel: [w1343 w1344] -> w1319
                      frame False {
                      }
                      frame True {
                        n232 = Multiply(x=w1345, y=-1.0) -> (x*y=w1344:dbl)
                      }
                    }
                    n233 = call "Motors Move Constant Velocity.vi"("Axis Multiplier"=w1316, "Axis"=w1315, "error in"=w1321, "VISA in"=w1318, "Speed (mm/s)"=w1319) -> ("error out"=w1320:errorcluster, "VISA out"=w1317:refnum<visa-resource-name>)  [unwired: 5 in]
                    n234 = while {
                      tunnel: w1317 -> [w1332]
                      tunnel: [w1334] -> w1325
                      tunnel: w1320 -> [w1335]
                      tunnel: [w1333] -> w1324
                      tunnel: w1316 -> [w1331]
                      tunnel: w1311 -> [w1330]
                      tunnel: w1310 -> [_]
                      tunnel: w1309 -> [_]
                      tunnel: w1308 -> [w1329]
                      tunnel: w1307 -> [w1328]
                      tunnel: w1306 -> [w1327]
                      stop <- w1340 continue-if-true
                      n235 = property on="Property Node" class="Bool (strict)"(reference=w1328) -> ("Value"=w1341:bool)  [unwired: 1 in, 2 out]
                      n236 = property on="Property Node" class="Bool (strict)"(reference=w1327) -> ("Value"=w1342:bool)  [unwired: 1 in, 2 out]
                      n237 = Or(x=w1341, y=w1342) -> (x .or. y?=w1340:bool)
                      n238 = call "Motors Status.vi"("error in"=w1335, "VISA in"=w1332, "Axis"=1, "Axis Multiplier"=w1331) -> ("error out"=w1333:errorcluster, "VISA out"=w1334:refnum<visa-resource-name>, "OS"=w1338:i32, "Actual Position (mm or deg)"=w1336:dbl)  [unwired: 3 in]
                      n239 = call "Motors Decipher Status.vi"("OS"=w1338) -> ("Status"=w1337:string)
                      n240 = property on="Property Node" class="DigNum (strict)"(reference=w1330, "Value"=w1336) -> ()  [unwired: 1 in, 2 out]
                      n241 = property on="Property Node" class="Str"(reference=w1329, "Value"=w1337) -> ()  [unwired: 1 in, 2 out]
                    }
                    n242 = call "Motors Stop.vi"("error in"=w1324, "Axis"=w1315, "VISA in"=w1325) -> ("error out"=w1322:errorcluster, "VISA out"=w1323:refnum<visa-resource-name>)
                  }
                }
              }
              frame #1 {
                n243 = property on="Property Node" class="Bool (strict)"(reference=w1348, "Value"=FALSE) -> ()  [unwired: 1 in, 2 out]
                n244 = property on="Property Node" class="Bool (strict)"(reference=w1347, "Value"=FALSE) -> ()  [unwired: 1 in, 2 out]
              }
            }
          }
        }
        n245 = property on="Property Node" class="Bool (strict)"() -> ("Value"=w305:bool)  [unwired: 2 in, 2 out]
        n246 = property on="Property Node" class="Bool (strict)"() -> ("Value"=w306:bool)  [unwired: 2 in, 2 out]
        n247 = case shown="True" w341 {
          tunnel: w343 -> [w1164 w1171]
          tunnel: w342 -> [w1163 w1170]
          tunnel: w196 -> [_ w1172]
          tunnel: [w1164 w1169] -> w340
          tunnel: [w1163 w1168] -> w339
          tunnel: w309 -> [_ w1167]
          frame False {
          }
          frame True {
            n248 = flat-sequence {
              tunnel: w1172 -> [w1178]
              tunnel: w1171 -> [w1177]
              tunnel: w1170 -> [w1176]
              tunnel: w1167 -> [w1173]
              tunnel: [w1175] -> w1166
              tunnel: [w1174] -> w1165
              tunnel: [w1232] -> w1168
              tunnel: [w1233] -> w1169
              tunnel: w1166 -> [w1233]
              tunnel: w1165 -> [w1232]
              frame #0 {
                n249 = case shown="False" w1178 {
                  tunnel: w1177 -> [w1184 w1204]
                  tunnel: w1176 -> [w1183 w1207]
                  tunnel: [w1182 w1211] -> w1175
                  tunnel: [w1181 w1210] -> w1174
                  tunnel: w1173 -> [w1180 w1209]
                  frame False {
                    n250 = property on="Property Node" class="Bool (strict)"() -> ("Value"=w1179:bool)  [unwired: 2 in, 2 out]
                    n251 = case shown="False" w1179 {
                      tunnel: w1184 -> [w1189 w1200]
                      tunnel: w1183 -> [w1194 w1199]
                      tunnel: [w1190 w1200] -> w1182
                      tunnel: [w1193 w1199] -> w1181
                      tunnel: w1180 -> [w1192 _]
                      frame False {
                        n252 = property on="Property Node" class="Bool (strict)"("Value"=TRUE ("Y Moving")) -> ()  [unwired: 2 in, 2 out]
                        n253 = case shown="True" w1192 {
                          tunnel: "Delta Y (mm)" -> [w1195 w1197]
                          tunnel: [w1195 w1196] -> w1188
                          frame False {
                          }
                          frame True {
                            n254 = Multiply(x=w1197, y=-1.0) -> (x*y=w1196:dbl)
                          }
                        }
                        n255 = property on="Property Node" class="DigNum (strict)"() -> ("Value"=w1186:u32)  [unwired: 2 in, 2 out]
                        n256 = call "Motors Move Relative.vi"("Axis Multiplier"=w1186, "Axis"=2, "error in"=w1194, "VISA in"=w1189, "Distance (mm)"=w1188) -> ("error out"=w1193:errorcluster, "VISA out"=w1190:refnum<visa-resource-name>)  [unwired: 5 in]
                      }
                      frame True {
                      }
                    }
                  }
                  frame True {
                    w1201 = 2 ("Axis")
                    n257 = case shown="True" w1209 {
                      tunnel: "Y Speed (mm/s)" -> [w1226 w1228]
                      tunnel: [w1226 w1227] -> w1205
                      frame False {
                      }
                      frame True {
                        n258 = Multiply(x=w1228, y=-1.0) -> (x*y=w1227:dbl)
                      }
                    }
                    n259 = property on="Property Node" class="DigNum (strict)"() -> ("Value"=w1202:u32)  [unwired: 2 in, 2 out]
                    n260 = call "Motors Move Constant Velocity.vi"("Axis Multiplier"=w1202, "Axis"=w1201, "error in"=w1207, "VISA in"=w1204, "Speed (mm/s)"=w1205) -> ("error out"=w1206:errorcluster, "VISA out"=w1203:refnum<visa-resource-name>)  [unwired: 5 in]
                    n261 = while {
                      tunnel: w1203 -> [w1216]
                      tunnel: [w1215] -> w1213
                      tunnel: w1206 -> [w1218]
                      tunnel: [w1217] -> w1212
                      tunnel: w1202 -> [w1214]
                      stop <- w1225 continue-if-true
                      n262 = property on="Property Node" class="Bool (strict)"() -> ("Value"=w1224:bool)  [unwired: 2 in, 2 out]
                      n263 = property on="Property Node" class="Bool (strict)"() -> ("Value"=w1223:bool)  [unwired: 2 in, 2 out]
                      n264 = Or(x=w1224, y=w1223) -> (x .or. y?=w1225:bool)
                      n265 = call "Motors Status.vi"("error in"=w1218, "VISA in"=w1216, "Axis"=2, "Axis Multiplier"=w1214) -> ("error out"=w1217:errorcluster, "VISA out"=w1215:refnum<visa-resource-name>, "OS"=w1220:i32, "Actual Position (mm or deg)"=w1221:dbl)  [unwired: 3 in]
                      n266 = property on="Property Node" class="DigNum (strict)"("Value"=w1221) -> ()  [unwired: 2 in, 2 out]
                      n267 = call "Motors Decipher Status.vi"("OS"=w1220) -> ("Status"=w1219:string)
                      n268 = property on="Property Node" class="Str"("Value"=w1219) -> ()  [unwired: 2 in, 2 out]
                    }
                    n269 = call "Motors Stop.vi"("error in"=w1212, "Axis"=w1201, "VISA in"=w1213) -> ("error out"=w1210:errorcluster, "VISA out"=w1211:refnum<visa-resource-name>)
                  }
                }
              }
              frame #1 {
                n270 = property on="Property Node" class="Bool (strict)"("Value"=FALSE) -> ()  [unwired: 2 in, 2 out]
                n271 = property on="Property Node" class="Bool (strict)"("Value"=FALSE) -> ()  [unwired: 2 in, 2 out]
              }
            }
          }
        }
        n272 = case shown="True" w338 {
          tunnel: w340 -> [w1050 w1069]
          tunnel: w339 -> [w1049 w1062]
          tunnel: w196 -> [_ w1070]
          tunnel: [w1050 w1068] -> w335
          tunnel: [w1049 w1067] -> w336
          tunnel: w308 -> [_ w1066]
          tunnel: w181 -> [_ w1063]
          tunnel: w180 -> [_ w1061]
          tunnel: w179 -> [_ w1060]
          tunnel: w170 -> [_ w1059]
          tunnel: w173 -> [_ w1058]
          tunnel: w172 -> [_ w1057]
          tunnel: w171 -> [_ w1056]
          tunnel: w170 -> [_ w1055]
          tunnel: w169 -> [_ w1054]
          tunnel: w168 -> [_ w1053]
          tunnel: w167 -> [_ w1052]
          tunnel: w166 -> [_ w1051]
          frame False {
          }
          frame True {
            n273 = flat-sequence {
              tunnel: w1070 -> [w1086]
              tunnel: w1069 -> [w1085]
              tunnel: w1066 -> [w1082]
              tunnel: [w1084] -> w1065
              tunnel: [w1083] -> w1064
              tunnel: w1063 -> [w1081]
              tunnel: w1062 -> [w1080]
              tunnel: w1061 -> [w1079]
              tunnel: w1060 -> [w1078]
              tunnel: w1059 -> [w1077]
              tunnel: w1058 -> [w1076]
              tunnel: w1057 -> [w1075]
              tunnel: w1056 -> [w1074]
              tunnel: w1053 -> [w1073]
              tunnel: w1052 -> [w1072]
              tunnel: w1051 -> [w1071]
              tunnel: [w1161] -> w1067
              tunnel: [w1162] -> w1068
              tunnel: w1065 -> [w1162]
              tunnel: w1064 -> [w1161]
              tunnel: w1055 -> [w1158]
              tunnel: w1054 -> [w1157]
              frame #0 {
                n274 = case shown="False" w1086 {
                  tunnel: w1085 -> [w1096 w1128]
                  tunnel: w1080 -> [w1095 w1131]
                  tunnel: [w1094 w1134] -> w1084
                  tunnel: [w1093 w1133] -> w1083
                  tunnel: w1082 -> [w1092 w1122]
                  tunnel: w1081 -> [_ w1125]
                  tunnel: w1080 -> [_ w1124]
                  tunnel: w1079 -> [_ w1121]
                  tunnel: w1078 -> [_ w1120]
                  tunnel: w1077 -> [_ w1119]
                  tunnel: w1076 -> [_ w1118]
                  tunnel: w1075 -> [_ w1117]
                  tunnel: w1074 -> [_ w1116]
                  tunnel: w1073 -> [w1090 _]
                  tunnel: w1072 -> [w1089 _]
                  tunnel: w1071 -> [w1087 _]
                  frame False {
                    n275 = property on="Property Node" class="Bool (strict)"(reference=w1090) -> (reference out=w1088:refnum<vi>, "Value"=w1091:bool)  [unwired: 1 in, 1 out]
                    n276 = case shown="False" w1091 {
                      tunnel: w1096 -> [w1102 w1115]
                      tunnel: w1095 -> [w1109 w1114]
                      tunnel: [w1103 w1115] -> w1094
                      tunnel: [w1108 w1114] -> w1093
                      tunnel: w1092 -> [w1107 _]
                      tunnel: w1089 -> [w1099 _]
                      tunnel: w1088 -> [w1098 _]
                      tunnel: w1087 -> [w1097 _]
                      frame False {
                        n277 = property on="Property Node" class="DigNum (strict)"(reference=w1097) -> ("Value"=w1105:u32)  [unwired: 1 in, 2 out]
                        n278 = property on="Property Node" class="DigNum (strict)"(reference=w1099) -> ("Value"=w1100:dbl)  [unwired: 1 in, 2 out]
                        n279 = property on="Property Node" class="Bool (strict)"(reference=w1098, "Value"=TRUE ("Z Moving")) -> ()  [unwired: 1 in, 2 out]
                        n280 = case shown="True" w1107 {
                          tunnel: w1100 -> [w1110 w1112]
                          tunnel: [w1110 w1111] -> w1104
                          frame False {
                          }
                          frame True {
                            n281 = Multiply(x=w1112, y=-1.0) -> (x*y=w1111:dbl)
                          }
                        }
                        n282 = call "Motors Move Relative.vi"("Axis Multiplier"=w1105, "Axis"=3, "error in"=w1109, "VISA in"=w1102, "Distance (mm)"=w1104) -> ("error out"=w1108:errorcluster, "VISA out"=w1103:refnum<visa-resource-name>)  [unwired: 5 in]
                      }
                      frame True {
                      }
                    }
                  }
                  frame True {
                    w1130 = 3 ("Axis")
                    n283 = property on="Property Node" class="DigNum (strict)"(reference=w1125) -> ("Value"=w1126:u32)  [unwired: 1 in, 2 out]
                    n284 = property on="Property Node" class="DigNum (strict)"(reference=w1121, error in=w1124) -> ("Value"=w1123:dbl)  [unwired: 2 out]
                    n285 = case shown="True" w1122 {
                      tunnel: w1123 -> [w1153 w1155]
                      tunnel: [w1153 w1154] -> w1129
                      frame False {
                      }
                      frame True {
                        n286 = Multiply(x=w1155, y=-1.0) -> (x*y=w1154:dbl)
                      }
                    }
                    n287 = call "Motors Move Constant Velocity.vi"("Axis Multiplier"=w1126, "Axis"=w1130, "error in"=w1131, "VISA in"=w1128, "Speed (mm/s)"=w1129) -> ("error out"=w1132:errorcluster, "VISA out"=w1127:refnum<visa-resource-name>)  [unwired: 5 in]
                    n288 = while {
                      tunnel: w1127 -> [w1143]
                      tunnel: [w1142] -> w1136
                      tunnel: w1132 -> [w1145]
                      tunnel: [w1144] -> w1135
                      tunnel: w1126 -> [w1141]
                      tunnel: w1120 -> [w1140]
                      tunnel: w1119 -> [_]
                      tunnel: w1118 -> [w1139]
                      tunnel: w1117 -> [w1138]
                      tunnel: w1116 -> [w1137]
                      stop <- w1152 continue-if-true
                      n289 = property on="Property Node" class="Bool (strict)"(reference=w1139) -> ("Value"=w1151:bool)  [unwired: 1 in, 2 out]
                      n290 = property on="Property Node" class="Bool (strict)"(reference=w1138) -> ("Value"=w1150:bool)  [unwired: 1 in, 2 out]
                      n291 = Or(x=w1151, y=w1150) -> (x .or. y?=w1152:bool)
                      n292 = call "Motors Status.vi"("error in"=w1145, "VISA in"=w1143, "Axis"=3, "Axis Multiplier"=w1141) -> ("error out"=w1144:errorcluster, "VISA out"=w1142:refnum<visa-resource-name>, "OS"=w1147:i32, "Actual Position (mm or deg)"=w1148:dbl)  [unwired: 3 in]
                      n293 = property on="Property Node" class="DigNum (strict)"(reference=w1140, "Value"=w1148) -> ()  [unwired: 1 in, 2 out]
                      n294 = call "Motors Decipher Status.vi"("OS"=w1147) -> ("Status"=w1146:string)
                      n295 = property on="Property Node" class="Str"(reference=w1137, "Value"=w1146) -> ()  [unwired: 1 in, 2 out]
                    }
                    n296 = call "Motors Stop.vi"("error in"=w1135, "Axis"=w1130, "VISA in"=w1136) -> ("error out"=w1133:errorcluster, "VISA out"=w1134:refnum<visa-resource-name>)
                  }
                }
              }
              frame #1 {
                n297 = property on="Property Node" class="Bool (strict)"(reference=w1158, "Value"=FALSE) -> ()  [unwired: 1 in, 2 out]
                n298 = property on="Property Node" class="Bool (strict)"(reference=w1157, "Value"=FALSE) -> ()  [unwired: 1 in, 2 out]
              }
            }
          }
        }
        n299 = Or(x=w306, y=w305) -> (x .or. y?=w337:bool)
        n300 = case shown="True" w337 {
          tunnel: w335 -> [w979 w986]
          tunnel: w336 -> [w978 w985]
          tunnel: w196 -> [_ w987]
          tunnel: [w979 w984] -> w334
          tunnel: [w978 w983] -> w327
          tunnel: w305 -> [_ w982]
          frame False {
          }
          frame True {
            n301 = flat-sequence {
              tunnel: w987 -> [w993]
              tunnel: w986 -> [w992]
              tunnel: w985 -> [w991]
              tunnel: w982 -> [w988]
              tunnel: [w990] -> w981
              tunnel: [w989] -> w980
              tunnel: [w1047] -> w983
              tunnel: [w1048] -> w984
              tunnel: w981 -> [w1048]
              tunnel: w980 -> [w1047]
              frame #0 {
                n302 = case shown="True" w993 {
                  tunnel: w992 -> [w999 w1020]
                  tunnel: w991 -> [w998 w1021]
                  tunnel: [w997 w1026] -> w990
                  tunnel: [w996 w1025] -> w989
                  tunnel: w988 -> [w995 w1024]
                  frame False {
                    n303 = property on="Property Node" class="Bool (strict)"() -> ("Value"=w994:bool)  [unwired: 2 in, 2 out]
                    n304 = case shown="False" w994 {
                      tunnel: w999 -> [w1002 w1015]
                      tunnel: w998 -> [w1009 w1014]
                      tunnel: [w1003 w1015] -> w997
                      tunnel: [w1008 w1014] -> w996
                      tunnel: w995 -> [w1007 _]
                      frame False {
                        n305 = property on="Property Node" class="Bool (strict)"("Value"=TRUE ("Theta Moving")) -> ()  [unwired: 2 in, 2 out]
                        n306 = case shown="True" w1007 {
                          tunnel: "Delta Theta (deg)" -> [w1010 w1012]
                          tunnel: [w1010 w1011] -> w1001
                          frame False {
                          }
                          frame True {
                            n307 = Multiply(x=w1012, y=-1.0) -> (x*y=w1011:dbl)
                          }
                        }
                        n308 = property on="Property Node" class="DigNum (strict)"() -> ("Value"=w1005:u32)  [unwired: 2 in, 2 out]
                        n309 = call "Motors Move Relative.vi"("Axis Multiplier"=w1005, "Axis"=4, "error in"=w1009, "VISA in"=w1002, "Distance (mm)"=w1001) -> ("error out"=w1008:errorcluster, "VISA out"=w1003:refnum<visa-resource-name>)  [unwired: 5 in]
                      }
                      frame True {
                      }
                    }
                  }
                  frame True {
                    w1018 = 4 ("Axis")
                    n310 = case shown="True" w1024 {
                      tunnel: "Theta Speed (deg/s)" -> [w1041 w1043]
                      tunnel: [w1041 w1042] -> w1016
                      frame False {
                      }
                      frame True {
                        n311 = Multiply(x=w1043, y=-1.0) -> (x*y=w1042:dbl)
                      }
                    }
                    n312 = property on="Property Node" class="DigNum (strict)"() -> ("Value"=w1017:u32)  [unwired: 2 in, 2 out]
                    n313 = call "Motors Move Constant Velocity.vi"("Axis Multiplier"=w1017, "Axis"=w1018, "error in"=w1021, "VISA in"=w1020, "Speed (mm/s)"=w1016) -> ("error out"=w1022:errorcluster, "VISA out"=w1019:refnum<visa-resource-name>)  [unwired: 5 in]
                    n314 = while {
                      tunnel: w1019 -> [w1031]
                      tunnel: [w1030] -> w1028
                      tunnel: w1022 -> [w1033]
                      tunnel: [w1032] -> w1027
                      tunnel: w1017 -> [w1029]
                      stop <- w1040 continue-if-true
                      n315 = property on="Property Node" class="Bool (strict)"() -> ("Value"=w1039:bool)  [unwired: 2 in, 2 out]
                      n316 = property on="Property Node" class="Bool (strict)"() -> ("Value"=w1038:bool)  [unwired: 2 in, 2 out]
                      n317 = Or(x=w1039, y=w1038) -> (x .or. y?=w1040:bool)
                      n318 = call "Motors Status.vi"("error in"=w1033, "VISA in"=w1031, "Axis"=4, "Axis Multiplier"=w1029) -> ("error out"=w1032:errorcluster, "VISA out"=w1030:refnum<visa-resource-name>, "OS"=w1035:i32, "Actual Position (mm or deg)"=w1036:dbl)  [unwired: 3 in]
                      n319 = property on="Property Node" class="DigNum (strict)"("Value"=w1036) -> ()  [unwired: 2 in, 2 out]
                      n320 = call "Motors Decipher Status.vi"("OS"=w1035) -> ("Status"=w1034:string)
                      n321 = property on="Property Node" class="Str"("Value"=w1034) -> ()  [unwired: 2 in, 2 out]
                    }
                    n322 = call "Motors Stop.vi"("error in"=w1027, "Axis"=w1018, "VISA in"=w1028) -> ("error out"=w1025:errorcluster, "VISA out"=w1026:refnum<visa-resource-name>)
                  }
                }
              }
              frame #1 {
                n323 = property on="Property Node" class="Bool (strict)"("Value"=FALSE) -> ()  [unwired: 2 in, 2 out]
                n324 = property on="Property Node" class="Bool (strict)"("Value"=FALSE) -> ()  [unwired: 2 in, 2 out]
              }
            }
          }
        }
        n325 = case shown="True" "X Set Slew Speed" {
          tunnel: [w969 w972] -> w331
          tunnel: w334 -> [w969 w973]
          tunnel: [w968 w976] -> w328
          tunnel: w327 -> [w968 w977]
          frame False {
          }
          frame True {
            n326 = property on="Property Node" class="Bool (strict)"("Value"=TRUE ("Need to Update Motor Parameters")) -> ()  [unwired: 2 in, 2 out]
            n327 = property on="Property Node" class="DigNum (strict)"() -> ("Value"=w970:u32)  [unwired: 2 in, 2 out]
            n328 = call "Motors Move Speed.vi"("Speed (mm or degree/sec)"="(mm/s)", "error in"=w977, "VISA in"=w973, "Axis"=u32 1, "Axis Multiplier"=w970) -> ("error out"=w976:errorcluster, "VISA out"=w972:refnum<visa-resource-name>)  [unwired: 5 in]
          }
        }
        n329 = case shown="True" "Y Set Slew Speed" {
          tunnel: [w959 w963] -> w332
          tunnel: w331 -> [w959 w960]
          tunnel: [w958 w966] -> w329
          tunnel: w328 -> [w958 w967]
          frame False {
          }
          frame True {
            n330 = property on="Property Node" class="Bool (strict)"("Value"=TRUE ("Need to Update Motor Parameters")) -> ()  [unwired: 2 in, 2 out]
            n331 = property on="Property Node" class="DigNum (strict)"() -> ("Value"=w961:u32)  [unwired: 2 in, 2 out]
            n332 = call "Motors Move Speed.vi"("Speed (mm or degree/sec)"="(mm/s) 3", "error in"=w967, "VISA in"=w960, "Axis"=u32 2, "Axis Multiplier"=w961) -> ("error out"=w966:errorcluster, "VISA out"=w963:refnum<visa-resource-name>)  [unwired: 5 in]
          }
        }
        n333 = case shown="True" "Z Set Slew Speed" {
          tunnel: [w949 w953] -> w333
          tunnel: w332 -> [w949 w952]
          tunnel: [w948 w956] -> w330
          tunnel: w329 -> [w948 w957]
          frame False {
          }
          frame True {
            n334 = property on="Property Node" class="Bool (strict)"("Value"=TRUE ("Need to Update Motor Parameters")) -> ()  [unwired: 2 in, 2 out]
            n335 = property on="Property Node" class="DigNum (strict)"() -> ("Value"=w950:u32)  [unwired: 2 in, 2 out]
            n336 = call "Motors Move Speed.vi"("Speed (mm or degree/sec)"="(mm/s) 2", "error in"=w957, "VISA in"=w952, "Axis"=u32 3, "Axis Multiplier"=w950) -> ("error out"=w956:errorcluster, "VISA out"=w953:refnum<visa-resource-name>)  [unwired: 5 in]
          }
        }
        n337 = case shown="True" "Theta Set Slew Speed" {
          tunnel: [w939 w943] -> w321
          tunnel: w333 -> [w939 w942]
          tunnel: [w938 w944] -> w322
          tunnel: w330 -> [w938 w947]
          frame False {
          }
          frame True {
            n338 = property on="Property Node" class="Bool (strict)"("Value"=TRUE ("Need to Update Motor Parameters")) -> ()  [unwired: 2 in, 2 out]
            n339 = property on="Property Node" class="DigNum (strict)"() -> ("Value"=w940:u32)  [unwired: 2 in, 2 out]
            n340 = call "Motors Move Speed.vi"("Speed (mm or degree/sec)"="(degrees/s)", "error in"=w947, "VISA in"=w942, "Axis"=u32 4, "Axis Multiplier"=w940) -> ("error out"=w944:errorcluster, "VISA out"=w943:refnum<visa-resource-name>)  [unwired: 5 in]
          }
        }
        n341 = Quotient & Remainder(x=w293, y=4) -> (x-y*floor(x/y)=w319:i32)  [unwired: 1 out]
        n342 = case shown="2" w319 {
          tunnel: w322 -> [w822 w836 w849 w864]
          tunnel: w321 -> [w823 w837 w851 w865]
          tunnel: [w821 w834 w848 w863] -> w316
          tunnel: [w820 w835 w850 w862] -> w315
          frame 0, Default {
            n343 = property on="Property Node" class="DigNum (strict)"() -> ("Value"=w819:u32)  [unwired: 2 in, 2 out]
            n344 = call "Motors Status.vi"("error in"=w822, "VISA in"=w823, "Axis"=1, "Axis Multiplier"=w819) -> ("error out"=w821:errorcluster, "VISA out"=w820:refnum<visa-resource-name>, "OS"=w829:i32, "Actual Position (mm or deg)"=w824:dbl)  [unwired: 3 in]
            n345 = property on="Property Node" class="DigNum (strict)"("Value"=w824) -> ()  [unwired: 2 in, 2 out]
            n346 = call "Motors Decipher Status.vi"("OS"=w829) -> ("Status"=w828:string)
            n347 = property on="Property Node" class="Str"("Value"=w828) -> ()  [unwired: 2 in, 2 out]
            n348 = Equal?(x=w828, y="Idle") -> (x = y?=w826:bool)
            n349 = case shown="False" w826 {
              tunnel: [TRUE FALSE] -> w825
              frame False {
              }
              frame True {
              }
            }
            n350 = property on="Property Node" class="Bool (strict)"("Value"=w825) -> ()  [unwired: 2 in, 2 out]
          }
          frame 1 {
            n351 = property on="Property Node" class="DigNum (strict)"() -> ("Value"=w833:u32)  [unwired: 2 in, 2 out]
            n352 = call "Motors Status.vi"("error in"=w836, "VISA in"=w837, "Axis"=2, "Axis Multiplier"=w833) -> ("error out"=w834:errorcluster, "VISA out"=w835:refnum<visa-resource-name>, "OS"=w842:i32, "Actual Position (mm or deg)"=w843:dbl)  [unwired: 3 in]
            n353 = property on="Property Node" class="DigNum (strict)"("Value"=w843) -> ()  [unwired: 2 in, 2 out]
            n354 = call "Motors Decipher Status.vi"("OS"=w842) -> ("Status"=w840:string)
            n355 = property on="Property Node" class="Str"("Value"=w840) -> ()  [unwired: 2 in, 2 out]
            n356 = Equal?(x=w840, y="Idle") -> (x = y?=w839:bool)
            n357 = case shown="False" w839 {
              tunnel: [TRUE FALSE] -> w838
              frame False {
              }
              frame True {
              }
            }
            n358 = property on="Property Node" class="Bool (strict)"("Value"=w838) -> ()  [unwired: 2 in, 2 out]
          }
          frame 2 {
            n359 = property on="Property Node" class="DigNum (strict)"() -> ("Value"=w847:u32)  [unwired: 2 in, 2 out]
            n360 = call "Motors Status.vi"("error in"=w849, "VISA in"=w851, "Axis"=3, "Axis Multiplier"=w847) -> ("error out"=w848:errorcluster, "VISA out"=w850:refnum<visa-resource-name>, "OS"=w856:i32, "Actual Position (mm or deg)"=w857:dbl)  [unwired: 3 in]
            n361 = property on="Property Node" class="DigNum (strict)"("Value"=w857) -> ()  [unwired: 2 in, 2 out]
            n362 = call "Motors Decipher Status.vi"("OS"=w856) -> ("Status"=w854:string)
            n363 = property on="Property Node" class="Str"("Value"=w854) -> ()  [unwired: 2 in, 2 out]
            n364 = Equal?(x=w854, y="Idle") -> (x = y?=w853:bool)
            n365 = case shown="False" w853 {
              tunnel: [TRUE FALSE] -> w852
              frame False {
              }
              frame True {
              }
            }
            n366 = property on="Property Node" class="Bool (strict)"("Value"=w852) -> ()  [unwired: 2 in, 2 out]
          }
          frame 3 {
            n367 = property on="Property Node" class="DigNum (strict)"() -> ("Value"=w861:u32)  [unwired: 2 in, 2 out]
            n368 = call "Motors Status.vi"("error in"=w864, "VISA in"=w865, "Axis"=4, "Axis Multiplier"=w861) -> ("error out"=w863:errorcluster, "VISA out"=w862:refnum<visa-resource-name>, "OS"=w870:i32, "Actual Position (mm or deg)"=w871:dbl)  [unwired: 3 in]
            n369 = property on="Property Node" class="DigNum (strict)"("Value"=w871) -> ()  [unwired: 2 in, 2 out]
            n370 = call "Motors Decipher Status.vi"("OS"=w870) -> ("Status"=w868:string)
            n371 = property on="Property Node" class="Str"("Value"=w868) -> ()  [unwired: 2 in, 2 out]
            n372 = Equal?(x=w868, y="Idle") -> (x = y?=w867:bool)
            n373 = case shown="True" w867 {
              tunnel: [TRUE FALSE] -> w866
              frame False {
              }
              frame True {
              }
            }
            n374 = property on="Property Node" class="Bool (strict)"("Value"=w866) -> ()  [unwired: 2 in, 2 out]
          }
        }
        n375 = case shown="True" "Go To Saved Position" {
          tunnel: w316 -> [w788 w790]
          tunnel: w315 -> [w787 w796]
          tunnel: [w788 w809] -> w314
          tunnel: [w787 w808] -> w313
          frame False {
          }
          frame True {
            w806 = 4 ("index (row)")
            w804 = 3 ("index (row)")
            w801 = 2 ("index (row)")
            w798 = 1 ("index (row)")
            n376 = property on="Property Node" class="Path"() -> ("Value"=w791:path)  [unwired: 2 in, 2 out]
            n377 = call "Motors Position Load.vi"("error in"=w790, "file path"=w791) -> ("error out"=w789:errorcluster, "Positions"=w813:string[][])
            n378 = property on="Property Node" class="DigNum (strict)"() -> ("Value"=w795:u32)  [unwired: 2 in, 2 out]
            n379 = Index Array(array=w813, index (row)=w806, index (col)="Defined Positions") -> (element=w814:string)
            n380 = Index Array(array=w813, index (row)=w804, index (col)="Defined Positions") -> (element=w815:string)
            n381 = Index Array(array=w813, index (row)=w801, index (col)="Defined Positions") -> (element=w817:string)
            n382 = Index Array(array=w813, index (row)=w798, index (col)="Defined Positions") -> (element=w818:string)
            n383 = Fract/Exp String To Number(string=w814) -> (number=w807:dbl)  [unwired: 3 in, 1 out]
            n384 = Fract/Exp String To Number(string=w815) -> (number=w803:dbl)  [unwired: 3 in, 1 out]
            n385 = Fract/Exp String To Number(string=w817) -> (number=w800:dbl)  [unwired: 3 in, 1 out]
            n386 = Fract/Exp String To Number(string=w818) -> (number=w797:dbl)  [unwired: 3 in, 1 out]
            n387 = property on="Property Node" class="DigNum (strict)"() -> ("Value"=w794:u32)  [unwired: 2 in, 2 out]
            n388 = property on="Property Node" class="DigNum (strict)"() -> ("Value"=w793:u32)  [unwired: 2 in, 2 out]
            n389 = call "Motors Move Absolute.vi"("Axis Multiplier"=w795, "Axis"=w798, "error in"=w789, "VISA in"=w796, "Position (mm or degree)"=w797) -> ("error out"=w816:errorcluster, "VISA out"=w799:refnum<visa-resource-name>)  [unwired: 5 in]
            n390 = property on="Property Node" class="DigNum (strict)"() -> ("Value"=w792:u32)  [unwired: 2 in, 2 out]
            n391 = call "Motors Move Absolute.vi"("Axis Multiplier"=w794, "Axis"=w801, "error in"=w816, "VISA in"=w799, "Position (mm or degree)"=w800) -> ("error out"=w812:errorcluster, "VISA out"=w802:refnum<visa-resource-name>)  [unwired: 5 in]
            n392 = call "Motors Move Absolute.vi"("Axis Multiplier"=w793, "Axis"=w804, "error in"=w812, "VISA in"=w802, "Position (mm or degree)"=w803) -> ("error out"=w811:errorcluster, "VISA out"=w805:refnum<visa-resource-name>)  [unwired: 5 in]
            n393 = call "Motors Move Absolute.vi"("Axis Multiplier"=w792, "Axis"=w806, "error in"=w811, "VISA in"=w805, "Position (mm or degree)"=w807) -> ("error out"=w809:errorcluster, "VISA out"=w808:refnum<visa-resource-name>)  [unwired: 5 in]
          }
        }
        n394 = property on="Property Node" class="Bool (strict)"() -> ("Value"=w320:bool)  [unwired: 2 in, 2 out]
        n395 = case shown="True" w320 {
          tunnel: w314 -> [w876 w879]
          tunnel: w313 -> [w875 w880]
          tunnel: [w875 w878] -> _
          tunnel: [w876 w877] -> w302
          frame False {
          }
          frame True {
            n396 = property on="Property Node" class="Bool (strict)"("Value"=FALSE ("Need to Update Motor Parameters")) -> ()  [unwired: 2 in, 2 out]
            n397 = flat-sequence {
              tunnel: w880 -> [w886]
              tunnel: w879 -> [w885]
              tunnel: [w884] -> w878
              tunnel: [w883] -> w877
              frame #0 {
                n398 = call <vilib>:"Set Busy.vi"() -> ()  [unwired: 10 in, 2 out]
                n399 = property on="Property Node" class="Str"("Value"="Updating Motor Parameters\nThis Should Take About 5 Seconds" ("Status Theta")) -> ()  [unwired: 2 in, 2 out]
              }
              frame #1 {
                n400 = call "Motors Status Verbose.vi"("Axis"=1, "VISA in"=w886, "error in"=w885) -> ("Slew Speed (mm or deg/s)"=w905:dbl, "Jogger Normal Speed (mm or deg/s)"=w906:dbl, "Jogger Fast Speed (mm or deg/s)"=w907:dbl, "Actual Position (mm or deg)"=w922:dbl, "OS"=w893:i32, "Mode"=w931:string, "VISA out"=w911:refnum<visa-resource-name>, "Creep Speed (mm or deg/s)"=w936:dbl, "error out"=w890:errorcluster)  [unwired: 4 in]
                n401 = property on="Property Node" class="Str"("Value"=w931) -> ()  [unwired: 2 in, 2 out]
                n402 = property on="Property Node" class="DigNum (strict)"("Value"=w905) -> ()  [unwired: 2 in, 2 out]
                n403 = property on="Property Node" class="DigNum (strict)"("Value"=w906) -> ()  [unwired: 2 in, 2 out]
                n404 = property on="Property Node" class="DigNum (strict)"("Value"=w907) -> ()  [unwired: 2 in, 2 out]
                n405 = property on="Property Node" class="DigNum (strict)"("Value"=w922) -> ()  [unwired: 2 in, 2 out]
                n406 = call "Motors Decipher Status.vi"("OS"=w893) -> ("Status"=w933:string)
                n407 = call "Motors Status Verbose.vi"("Axis"=2, "VISA in"=w911, "error in"=w890) -> ("Slew Speed (mm or deg/s)"=w908:dbl, "Jogger Normal Speed (mm or deg/s)"=w909:dbl, "Jogger Fast Speed (mm or deg/s)"=w910:dbl, "Actual Position (mm or deg)"=w923:dbl, "OS"=w894:i32, "Mode"=w932:string, "VISA out"=w912:refnum<visa-resource-name>, "Creep Speed (mm or deg/s)"=w901:dbl, "error out"=w891:errorcluster)  [unwired: 4 in]
                n408 = property on="(mm/s)" class="DigNum (strict)"("Minimum"=w936) -> ()  [unwired: 2 in, 2 out]
                n409 = property on="Property Node" class="Str"("Value"=w933) -> ()  [unwired: 2 in, 2 out]
                n410 = property on="Property Node" class="Str"("Value"=w932) -> ()  [unwired: 2 in, 2 out]
                n411 = property on="Property Node" class="DigNum (strict)"("Value"=w908) -> ()  [unwired: 2 in, 2 out]
                n412 = property on="Property Node" class="DigNum (strict)"("Value"=w909) -> ()  [unwired: 2 in, 2 out]
                n413 = property on="Property Node" class="DigNum (strict)"("Value"=w910) -> ()  [unwired: 2 in, 2 out]
                n414 = property on="Property Node" class="DigNum (strict)"("Value"=w923) -> ()  [unwired: 2 in, 2 out]
                n415 = call "Motors Decipher Status.vi"("OS"=w894) -> ("Status"=w924:string)
                n416 = call "Motors Status Verbose.vi"("Axis"=3, "VISA in"=w912, "error in"=w891) -> ("Slew Speed (mm or deg/s)"=w921:dbl, "Jogger Normal Speed (mm or deg/s)"=w920:dbl, "Jogger Fast Speed (mm or deg/s)"=w919:dbl, "Actual Position (mm or deg)"=w918:dbl, "OS"=w895:i32, "Mode"=w925:string, "VISA out"=w913:refnum<visa-resource-name>, "Creep Speed (mm or deg/s)"=w902:dbl, "error out"=w892:errorcluster)  [unwired: 4 in]
                n417 = property on="(mm/s) 3" class="DigNum (strict)"("Minimum"=w901) -> ()  [unwired: 2 in, 2 out]
                n418 = Not Equal?(x=w933, y="Idle") -> (x != y?=w914:bool)
                n419 = property on="Property Node" class="Str"("Value"=w924) -> ()  [unwired: 2 in, 2 out]
                n420 = property on="Property Node" class="Str"("Value"=w925) -> ()  [unwired: 2 in, 2 out]
                n421 = property on="Property Node" class="DigNum (strict)"("Value"=w921) -> ()  [unwired: 2 in, 2 out]
                n422 = property on="Property Node" class="DigNum (strict)"("Value"=w920) -> ()  [unwired: 2 in, 2 out]
                n423 = property on="Property Node" class="DigNum (strict)"("Value"=w919) -> ()  [unwired: 2 in, 2 out]
                n424 = property on="Property Node" class="DigNum (strict)"("Value"=w918) -> ()  [unwired: 2 in, 2 out]
                n425 = property on="Property Node" class="Bool (strict)"("Value"=w914) -> ()  [unwired: 2 in, 2 out]
                n426 = property on="(mm/s) 2" class="DigNum (strict)"("Minimum"=w902) -> ()  [unwired: 2 in, 2 out]
                n427 = call "Motors Status Verbose.vi"("Axis"=4, "VISA in"=w913, "error in"=w892) -> ("Slew Speed (mm or deg/s)"=w927:dbl, "Jogger Normal Speed (mm or deg/s)"=w928:dbl, "Jogger Fast Speed (mm or deg/s)"=w929:dbl, "Actual Position (mm or deg)"=w930:dbl, "OS"=w896:i32, "Mode"=w934:string, "VISA out"=w884:refnum<visa-resource-name>, "Creep Speed (mm or deg/s)"=w903:dbl, "error out"=w883:errorcluster)  [unwired: 4 in]
                n428 = call "Motors Decipher Status.vi"("OS"=w895) -> ("Status"=w926:string)
                n429 = Not Equal?(x=w924, y="Idle") -> (x != y?=w915:bool)
                n430 = property on="Property Node" class="DigNum (strict)"("Value"=w927) -> ()  [unwired: 2 in, 2 out]
                n431 = property on="Property Node" class="DigNum (strict)"("Value"=w928) -> ()  [unwired: 2 in, 2 out]
                n432 = property on="Property Node" class="DigNum (strict)"("Value"=w929) -> ()  [unwired: 2 in, 2 out]
                n433 = property on="Property Node" class="DigNum (strict)"("Value"=w930) -> ()  [unwired: 2 in, 2 out]
                n434 = property on="Property Node" class="Str"("Value"=w926) -> ()  [unwired: 2 in, 2 out]
                n435 = property on="Property Node" class="Str"("Value"=w934) -> ()  [unwired: 2 in, 2 out]
                n436 = property on="(degrees/s)" class="DigNum (strict)"("Minimum"=w903) -> ()  [unwired: 2 in, 2 out]
                n437 = call "Motors Decipher Status.vi"("OS"=w896) -> ("Status"=w935:string)
                n438 = property on="Property Node" class="Bool (strict)"("Value"=w915) -> ()  [unwired: 2 in, 2 out]
                n439 = property on="Property Node" class="Str"("Value"=w935) -> ()  [unwired: 2 in, 2 out]
                n440 = Not Equal?(x=w926, y="Idle") -> (x != y?=w916:bool)
                n441 = Not Equal?(x=w935, y="Idle") -> (x != y?=w917:bool)
                n442 = property on="Property Node" class="Bool (strict)"("Value"=w916) -> ()  [unwired: 2 in, 2 out]
                n443 = property on="Property Node" class="Bool (strict)"("Value"=w917) -> ()  [unwired: 2 in, 2 out]
              }
              frame #2 {
                n444 = call <vilib>:"Unset Busy.vi"() -> ()  [unwired: 11 in, 1 out]
                n445 = property on="Property Node" class="Str"("Value"="Running" ("Status Theta")) -> ()  [unwired: 2 in, 2 out]
              }
            }
          }
        }
        n446 = property on="Property Node" class="Clust (strict)"("Value"=w302) -> ()  [unwired: 2 in, 2 out]
        "Loop i" <- w293
      }
    }
  }
  n447 = property on="Property Node" class="Bool (strict)"(reference=w54, "Value"=w71) -> ()  [unwired: 1 in, 2 out]
